vi "Autonomous Independent.vi"   [LabVIEW 2017]
doc: "This VI is called when autonomous begins, and will automatically be terminated when autonomous ends. You can carry out timed or sensor driven robot movement independently without needing to return to the caller."
uses:
  <vilib>/Rock Robotics/WPI/Utilities/WPI_GetSetVariantRefNum.vi
  <vilib>/Rock Robotics/Network Tables/NT Read String.vi
  <vilib>/Rock Robotics/Network Tables/NT Write Numeric Array.vi
  <vilib>/Rock Robotics/WPI/RobotDrive/WPI_RobotDriveArcadeDrive_Standard(NoSaturation).vi
panel:
  # "Be sure to right-click and choose Data Operations>>Make Current Value default if you want to save the array values with the VI"
types:
  T1 = typedef "WPI_JoystickDevRef.ctl" = cluster{"Device":T2}
  T2 = typedef "WPI_JoystickDeviceEnum.ctl" = enum16{"USB 0", "USB 1", "USB 2", "USB 3", "USB 4", "USB 5"}
  T3 = typedef "WPI_RobotDriveDevRef.ctl" = cluster{"DevStatus":errorcluster, "Motors[]":T4[], "Square Inputs":bool, "Max Output":dbl}
  T4 = typedef "WPI_MotorControlDeviceRef.ctl" = cluster{"DeviceStatus":errorcluster, "Type":T5, "PWM":cluster{"PWM Channel":T6, "DeadBand":T7}, "CAN":cluster{"Device Number":u8, "SetOutput VI Ref":variant, "GetOutput VI Ref":variant, "Enable VI Ref":variant, "Disable VI Ref":variant, "Data":variant}, "Invert":bool, "DIO PWM":cluster{"PWM \"Enable\" Channel":T6, "DIOChannel":T8, "PWM Rate":dbl}}
  T5 = typedef "WPI_MotorControlType.ctl" = enum16{"PWM", "CAN", "DIO PWM"}
  T6 = typedef "FPGA_DIOPWMChannel.ctl" = enum8{"PWM 0", "PWM 1", "PWM 2", "PWM 3", "PWM 4", "PWM 5", "PWM 6", "PWM 7", "PWM 8", "PWM 9", "PWM MXP 0", "PWM MXP 1", "PWM MXP 2", "PWM MXP 3", "PWM MXP 4", "PWM MXP 5", "PWM MXP 6", "PWM MXP 7", "PWM MXP 8", "PWM MXP 9", "Invalid"}
  T7 = typedef "WPI_PWMDeadband.ctl" = cluster{"Name":string, "maxPositivePwm":i32, "minPositivePwm":i32, "centerPwm":i32, "maxNegativePwm":i32, "minNegativePwm":i32, "angularRange":u16}
  T8 = typedef "FPGA_DIOChannel.ctl" = enum8{"DIO 0", "DIO 1", "DIO 2", "DIO 3", "DIO 4", "DIO 5", "DIO 6", "DIO 7", "DIO 8", "DIO 9", "DIO MXP 0", "DIO MXP 1", "DIO MXP 2", "DIO MXP 3", "DIO MXP 4", "DIO MXP 5", "DIO MXP 6", "DIO MXP 7", "DIO MXP 8", "DIO MXP 9", "DIO MXP 10", "DIO MXP 11", "DIO MXP 12", "DIO MXP 13", "DIO MXP 14", "DIO MXP 15", "SPI Port CS1", "SPI Port CS2", "SPI Port CS3", "SPI Port MISO", "SPI Port MOSI", "Invalid"}
  T9 = typedef "WPI_SwitchDevRef.ctl" = cluster{"DevStatus":errorcluster, "DIO Channel":T8, "CntIndex":T10, "Normally Closed":bool}
  T10 = typedef "FPGA_CounterCtrSystemIndex.ctl" = enum8{"Ctr 0", "Ctr 1", "Ctr 2", "Ctr 3", "Ctr 4", "Ctr 5", "Ctr 6", "Ctr 7", "Invalid"}
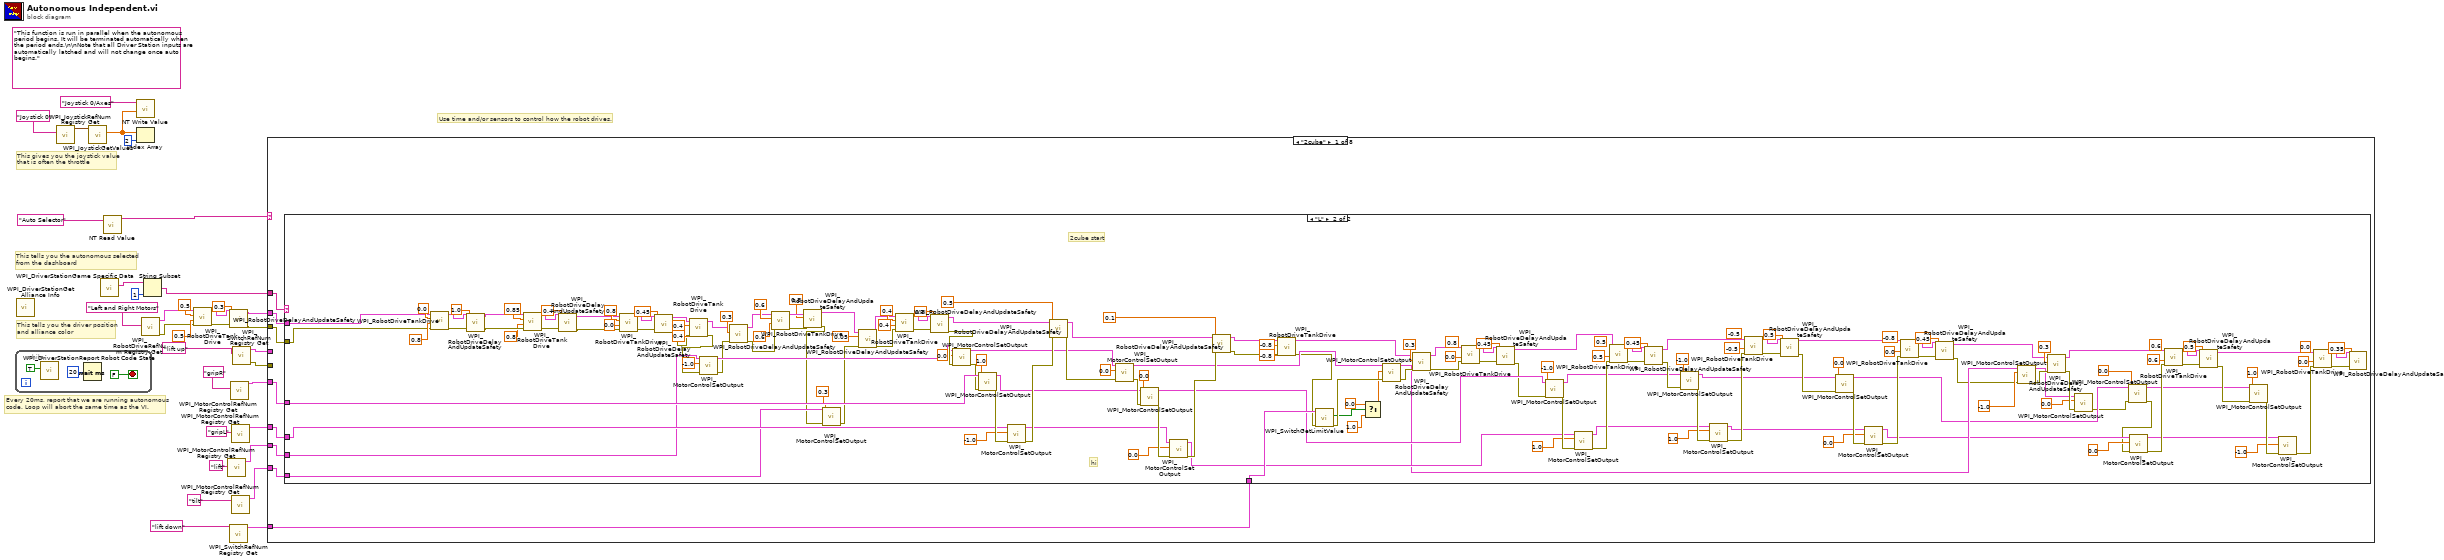
[diagram p0: block diagram]
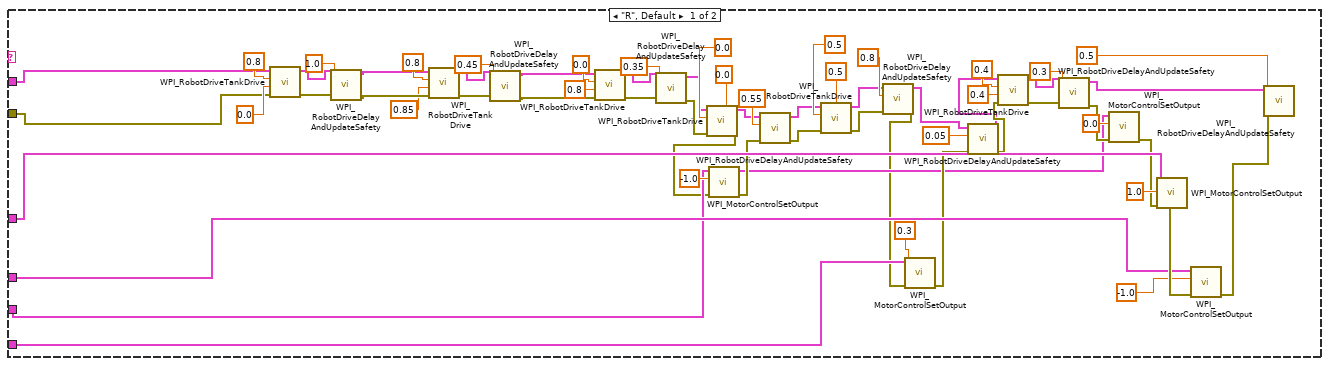
[diagram p2: hidden frame]
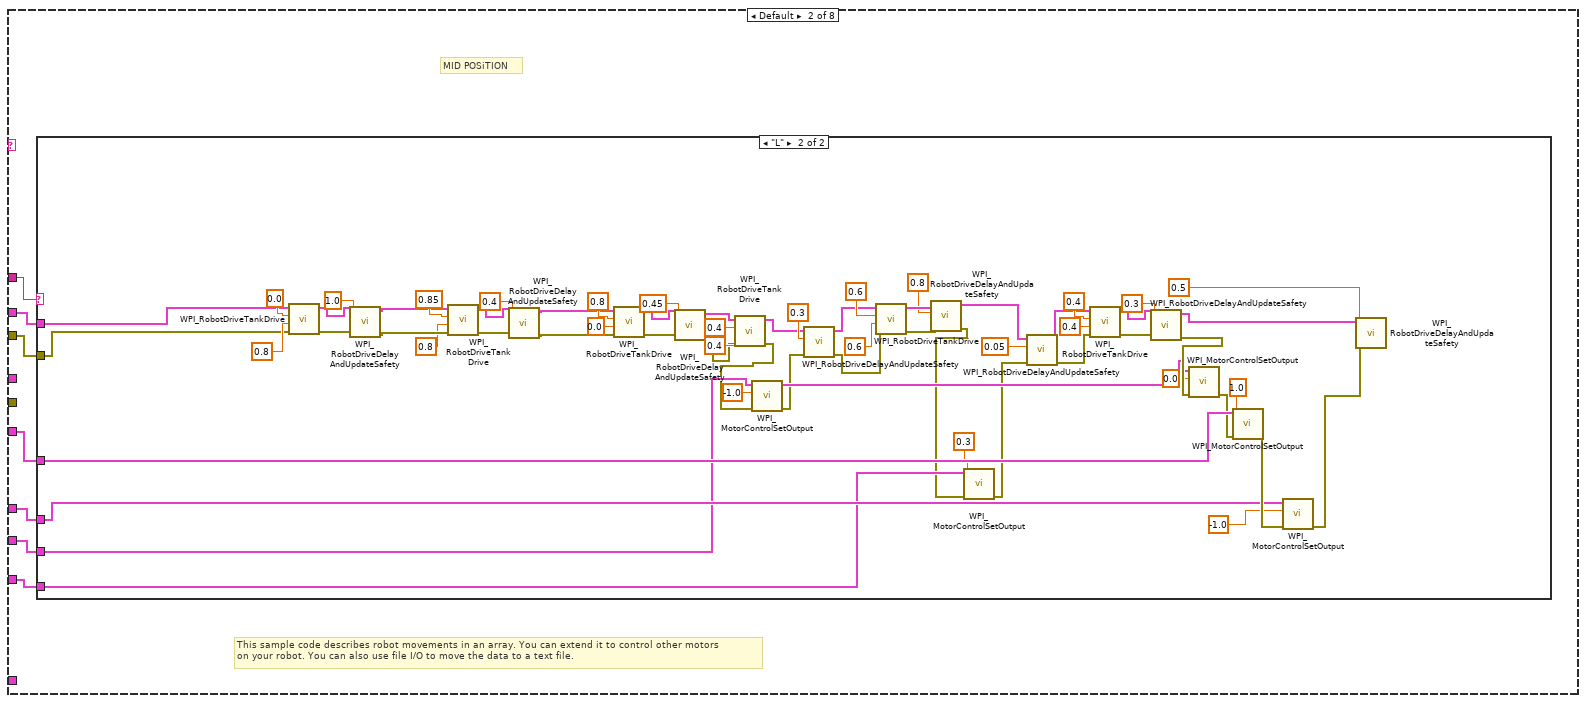
[diagram p3: hidden frame]
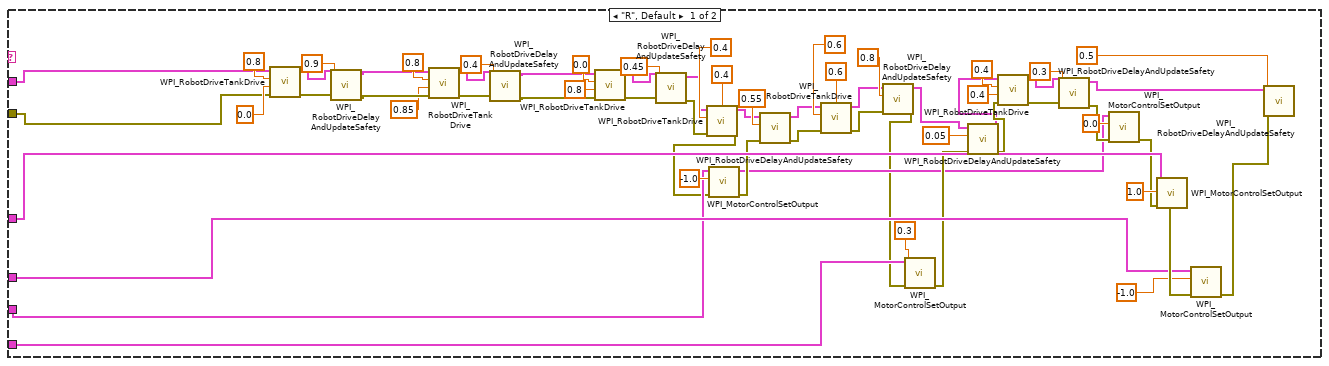
[diagram p4: hidden frame]
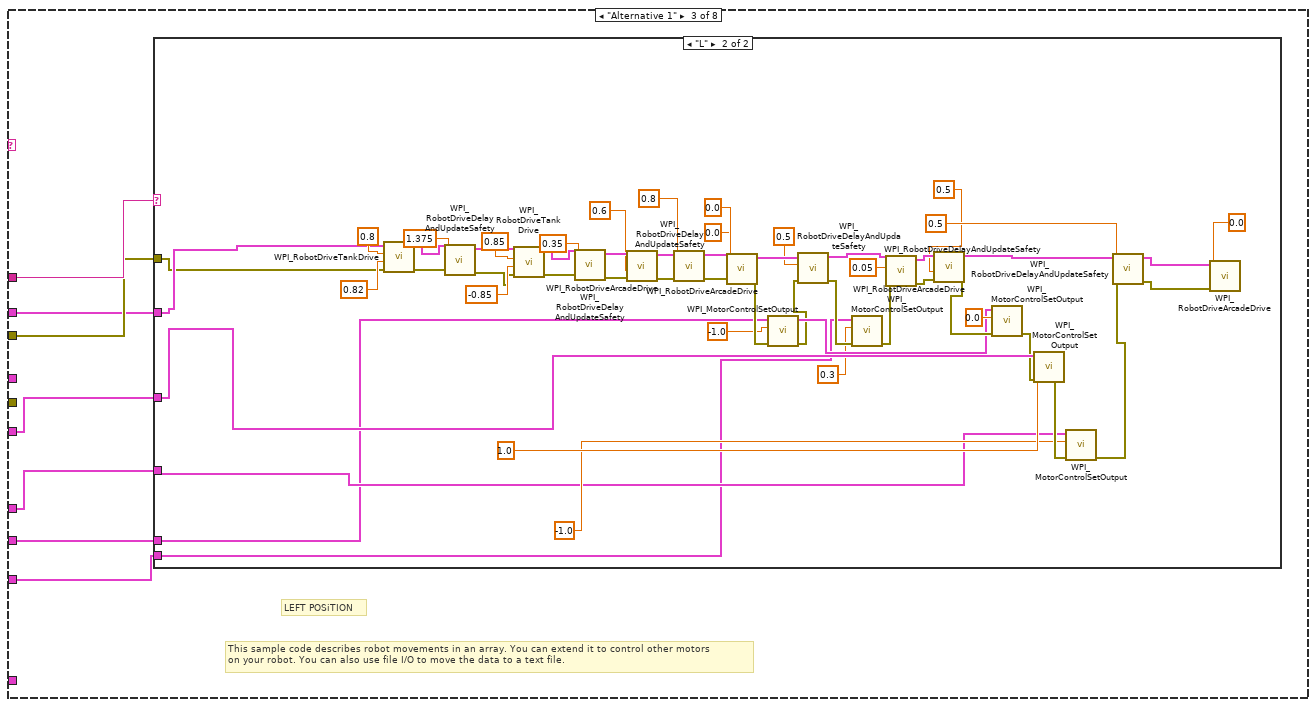
[diagram p5: hidden frame]
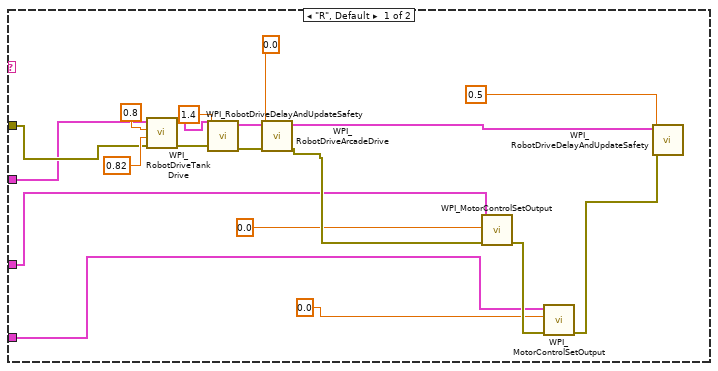
[diagram p6: hidden frame]
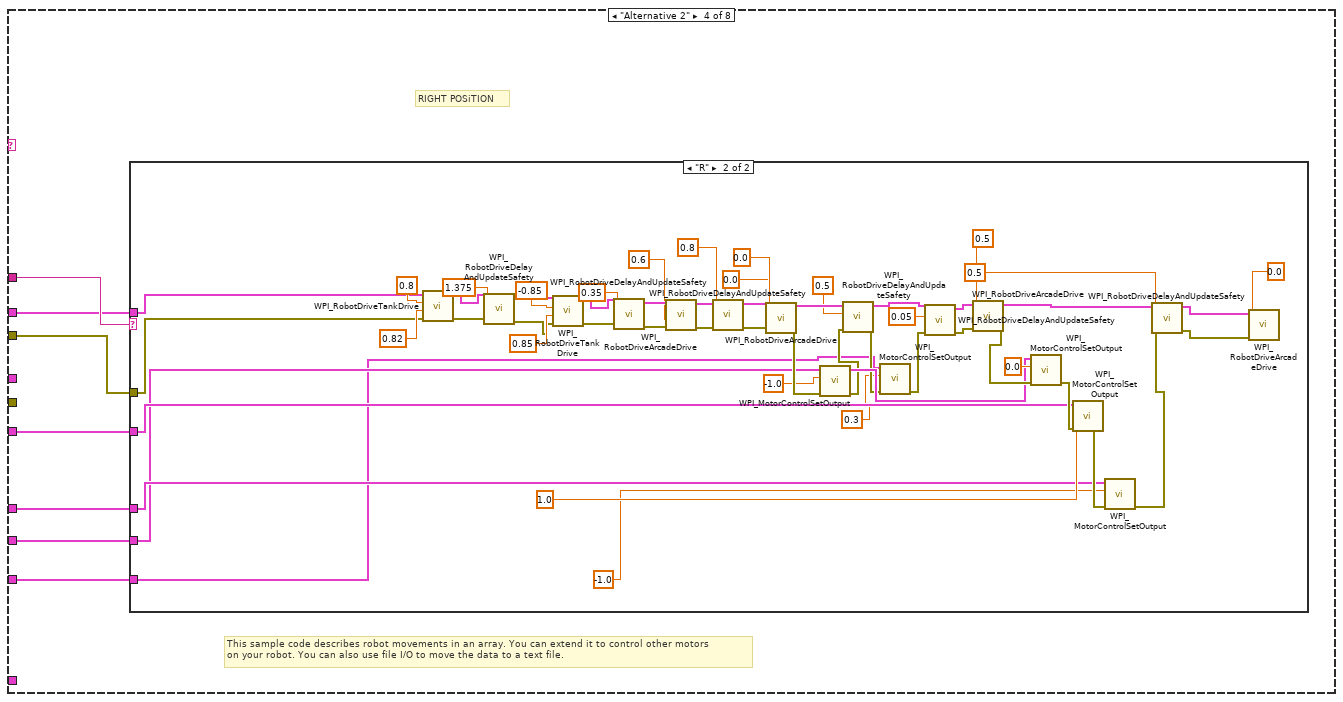
[diagram p7: hidden frame]
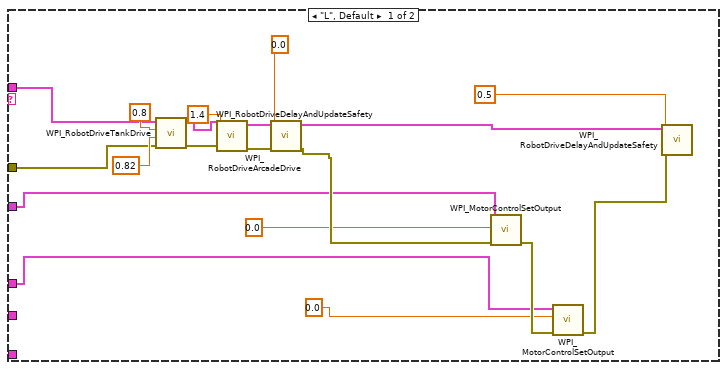
[diagram p8: hidden frame]
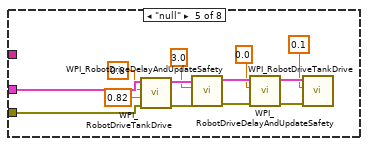
[diagram p9: hidden frame]
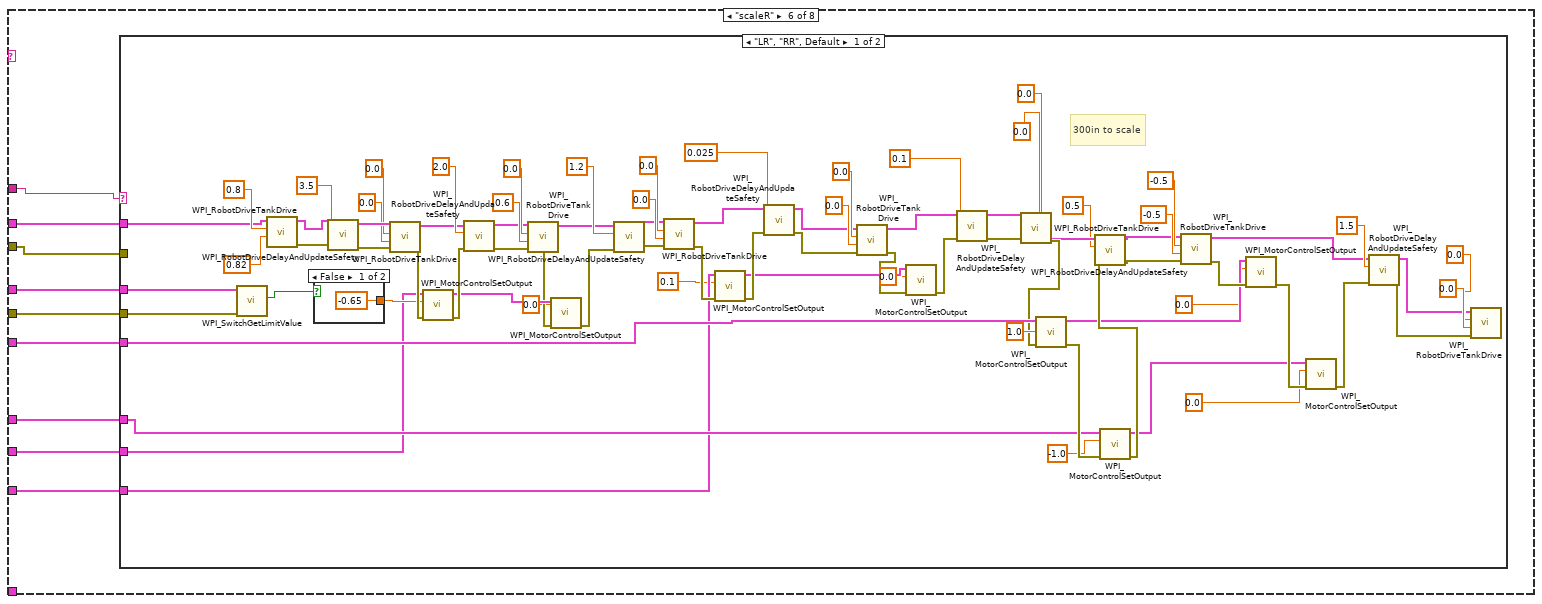
[diagram p10: hidden frame]
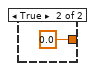
[diagram p11: hidden frame]
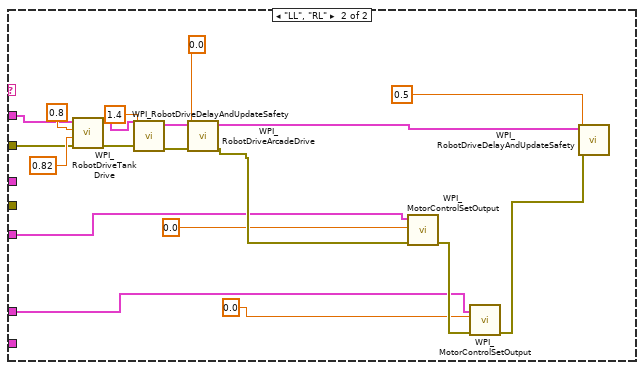
[diagram p12: hidden frame]
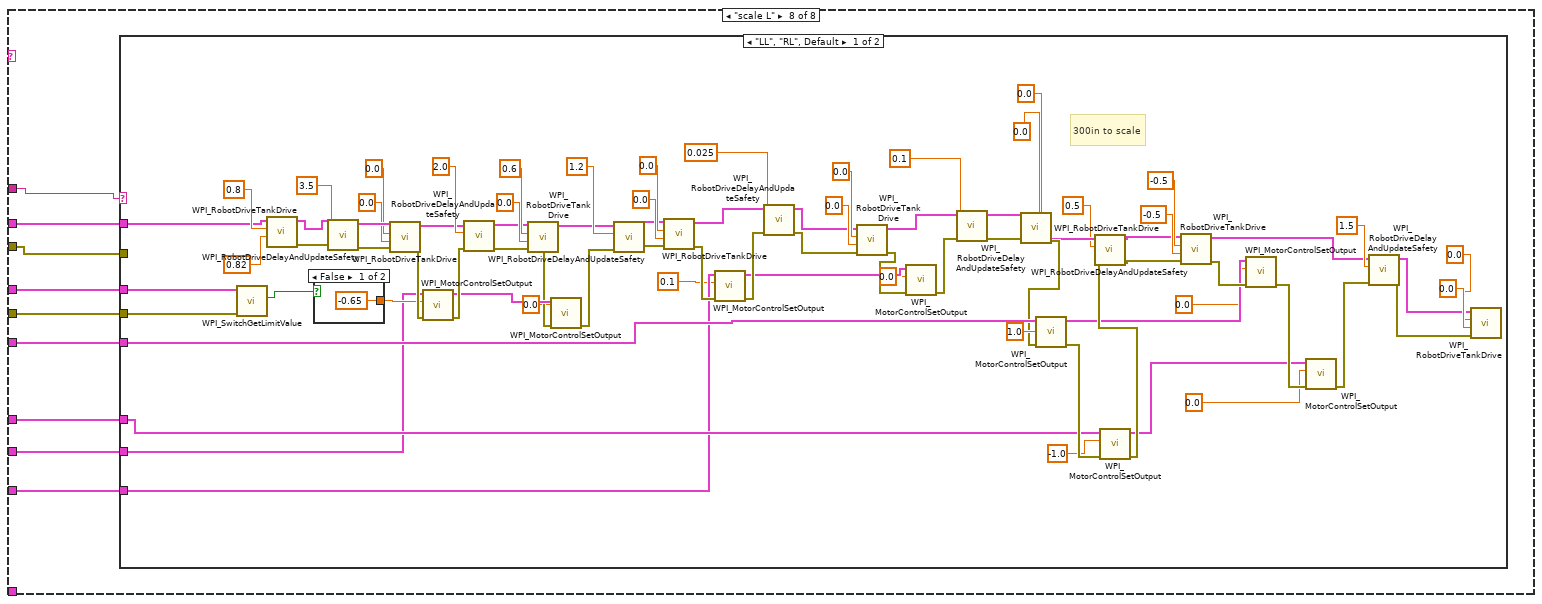
[diagram p14: hidden frame]
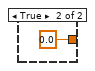
[diagram p15: hidden frame]
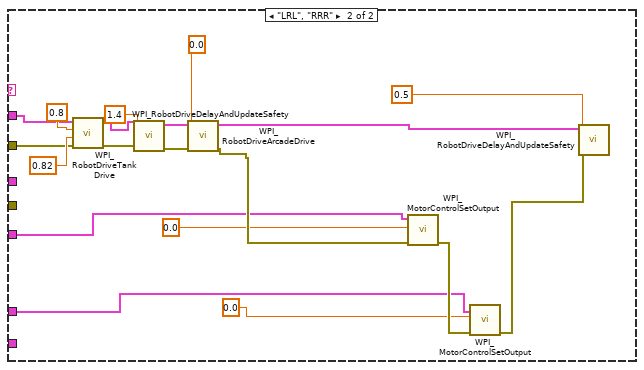
[diagram p16: hidden frame]
diagram:
  (unwired) "This function is run in parallel when the autonomous period begins. It will be terminated automatically when the period ends.\n\nNote that all Driver Station inputs are automatically latched and will not change once auto begins."
  # "This tells you the autonomous selected\nfrom the dashboard"
  # "Every 20ms, report that we are running autonomous\ncode. Loop will abort the same time as the VI."
  # "This gives you the joystick value\nthat is often the throttle"
  # "Use time and/or sensors to control how the robot drives."
  # "This tells you the driver position\nand alliance color"
  n1 = while {
    stop <- FALSE stop-if-true
    n2 = call <vilib>:"WPI_DriverStationReport Robot Code State.vi"("Autonomous"=TRUE) -> ()  [unwired: 10 in, 1 out]
    n3 = Wait (ms)(milliseconds to wait=u32 20) -> ()  [unwired: 1 out]
  }
  n4 = call <vilib>:"WPI_DriverStationGet Alliance Info.vi"() -> ()  [unwired: 12 out]
  n5 = call <vilib>:"WPI_JoystickRefNum Registry Get.vi"("refnum name"="Joystick 0") -> ("JoystickDevRef"=w32:T1)  [unwired: 1 in, 9 out]
  n6 = call <vilib>:"WPI_JoystickGetValues.vi"("JoystickDevRef"=w32) -> ("Axes"=w28:dbl[])  [unwired: 6 in, 4 out]
  n7 = call <vilib>:"WPI_DriverStationGame Specific Data.vi"() -> ("Game Specific Data"=w26:string)  [unwired: 11 in]
  n8 = call-poly <vilib>:"NT Read Value.vi"("Name"="Auto Selector") -> ("String"=w29:string)  [unwired: 9 in, 1 out]
  n9 = call-poly <vilib>:"NT Write Value.vi"("Numeric Array"=w28, "Name"="Joystick 0/Axes") -> ()  [unwired: 9 in, 1 out]
  n10 = Index Array(array=w28, index=2) -> ()  [unwired: 1 out]
  n11 = call <vilib>:"WPI_RobotDriveRefNum Registry Get.vi"("refnum name"="Left and Right Motors") -> ("error out"=w8:errorcluster, "RobotDriveDevRef"=w7:T3)  [unwired: 1 in, 8 out]
  n12 = String Subset(string=w26, length (rest)=1 ("length (rest)")) -> (substring=w24:string)  [unwired: 1 in]
  n13 = call <vilib>:"WPI_RobotDriveTankDrive.vi"("error in (no error)"=w8, "Right axis value"=0.5 ("Y axis value"), "Left axis value"=0.5 ("X axis value"), "RobotDriveDevRef"=w7) -> ("error out"=w12:errorcluster, "RobotDriveDevRef"=w11:T3)  [unwired: 5 in, 1 out]
  n14 = call <vilib>:"WPI_MotorControlRefNum Registry Get.vi"("refnum name"="lift") -> ("MotorControlDevRef"=w14:T4)  [unwired: 9 in, 1 out]
  n15 = call <vilib>:"WPI_RobotDriveDelayAndUpdateSafety.vi"("error in (no error)"=w12, "Delay (s)"=0.3, "RobotDriveDevRef"=w11) -> ("error out"=w5:errorcluster, "RobotDriveDevRef 2"=w6:T3)  [unwired: 7 in]
  n16 = call <vilib>:"WPI_SwitchRefNum Registry Get.vi"("refnum name"="lift down") -> ("SwitchDevRef"=w1:T9)  [unwired: 9 in, 1 out]
  n17 = call <vilib>:"WPI_MotorControlRefNum Registry Get.vi"("refnum name"="gripR") -> ("MotorControlDevRef"=w21:T4)  [unwired: 9 in, 1 out]
  n18 = call <vilib>:"WPI_MotorControlRefNum Registry Get.vi"("refnum name"="gripL") -> ("MotorControlDevRef"=w19:T4)  [unwired: 9 in, 1 out]
  n19 = call <vilib>:"WPI_MotorControlRefNum Registry Get.vi"("refnum name"="tilt") -> ("MotorControlDevRef"=w4:T4)  [unwired: 9 in, 1 out]
  n20 = call <vilib>:"WPI_SwitchRefNum Registry Get.vi"("refnum name"="lift up") -> ("error out"=w16:errorcluster, "SwitchDevRef"=w15:T9)  [unwired: 9 in]
  n21 = case shown="\"2cube\"" w29 {
    tunnel: w24 -> [w44 w279 w412 w492 _ w587 _ w696]
    tunnel: w5 -> [w42 w278 w411 w491 w575 w580 _ w689]
    tunnel: w21 -> [w41 w277 w410 w490 _ w584 _ w693]
    tunnel: w19 -> [w40 w276 w409 w489 _ w585 _ w694]
    tunnel: w6 -> [w43 w275 w408 w488 w576 w586 _ w695]
    tunnel: w16 -> [_ _ _ _ _ w583 _ w692]
    tunnel: w15 -> [_ _ _ _ _ w582 _ w691]
    tunnel: w14 -> [w39 w274 w407 w487 _ w581 _ w690]
    tunnel: w4 -> [w38 w273 w406 w486 _ w579 _ w688]
    tunnel: w1 -> [w37 _ _ _ _ _ _ _]
    frame "2cube" {
      n22 = case shown="\"L\"" w44 {
        tunnel: w42 -> [w97 w242]
        tunnel: w41 -> [w96 w241]
        tunnel: w40 -> [w95 w240]
        tunnel: w43 -> [w74 w239]
        tunnel: w39 -> [w64 w234]
        tunnel: w38 -> [w63 w229]
        tunnel: w37 -> [_ w189]
        frame "R", Default {
          n23 = call <vilib>:"WPI_RobotDriveTankDrive.vi"("error in (no error)"=w97, "Right axis value"=0.0 ("Y axis value"), "Left axis value"=0.8 ("X axis value"), "RobotDriveDevRef"=w74) -> ("error out"=w103:errorcluster, "RobotDriveDevRef"=w102:T3)  [unwired: 5 in, 1 out]
          n24 = call <vilib>:"WPI_RobotDriveDelayAndUpdateSafety.vi"("error in (no error)"=w103, "Delay (s)"=1.0, "RobotDriveDevRef"=w102) -> ("error out"=w89:errorcluster, "RobotDriveDevRef 2"=w90:T3)  [unwired: 7 in]
          n25 = call <vilib>:"WPI_RobotDriveTankDrive.vi"("error in (no error)"=w89, "Right axis value"=0.85, "Left axis value"=0.8 ("X axis value"), "RobotDriveDevRef"=w90) -> ("error out"=w93:errorcluster, "RobotDriveDevRef"=w92:T3)  [unwired: 5 in, 1 out]
          n26 = call <vilib>:"WPI_RobotDriveDelayAndUpdateSafety.vi"("error in (no error)"=w93, "Delay (s)"=0.45, "RobotDriveDevRef"=w92) -> ("error out"=w82:errorcluster, "RobotDriveDevRef 2"=w83:T3)  [unwired: 7 in]
          n27 = call <vilib>:"WPI_RobotDriveTankDrive.vi"("error in (no error)"=w82, "Right axis value"=0.8, "Left axis value"=0.0 ("X axis value"), "RobotDriveDevRef"=w83) -> ("error out"=w86:errorcluster, "RobotDriveDevRef"=w85:T3)  [unwired: 5 in, 1 out]
          n28 = call <vilib>:"WPI_RobotDriveDelayAndUpdateSafety.vi"("error in (no error)"=w86, "Delay (s)"=0.35, "RobotDriveDevRef"=w85) -> ("error out"=w51:errorcluster, "RobotDriveDevRef 2"=w52:T3)  [unwired: 7 in]
          n29 = call <vilib>:"WPI_RobotDriveTankDrive.vi"("error in (no error)"=w51, "Right axis value"=0.0 ("Y axis value"), "Left axis value"=0.0 ("X axis value"), "RobotDriveDevRef"=w52) -> ("error out"=w50:errorcluster, "RobotDriveDevRef"=w49:T3)  [unwired: 5 in, 1 out]
          n30 = call <vilib>:"WPI_MotorControlSetOutput.vi"("error in (no error)"=w50, "Output"=-1.0, "MotorControlDevRef"=w64) -> ("error out"=w67:errorcluster, "MotorControlDevRef"=w62:T4)  [unwired: 6 in, 1 out]
          n31 = call <vilib>:"WPI_RobotDriveDelayAndUpdateSafety.vi"("error in (no error)"=w67, "Delay (s)"=0.55 ("Output"), "RobotDriveDevRef"=w49) -> ("error out"=w48:errorcluster, "RobotDriveDevRef 2"=w47:T3)  [unwired: 7 in]
          n32 = call <vilib>:"WPI_RobotDriveTankDrive.vi"("error in (no error)"=w48, "Right axis value"=0.5 ("Y axis value"), "Left axis value"=0.5 ("X axis value"), "RobotDriveDevRef"=w47) -> ("error out"=w57:errorcluster, "RobotDriveDevRef"=w58:T3)  [unwired: 5 in, 1 out]
          n33 = call <vilib>:"WPI_RobotDriveDelayAndUpdateSafety.vi"("error in (no error)"=w57, "Delay (s)"=0.8, "RobotDriveDevRef"=w58) -> ("error out"=w45:errorcluster, "RobotDriveDevRef 2"=w46:T3)  [unwired: 7 in]
          n34 = call <vilib>:"WPI_MotorControlSetOutput.vi"("error in (no error)"=w45, "Output"=0.3, "MotorControlDevRef"=w63) -> ("error out"=w66:errorcluster)  [unwired: 6 in, 2 out]
          n35 = call <vilib>:"WPI_RobotDriveDelayAndUpdateSafety.vi"("error in (no error)"=w66, "Delay (s)"=0.05, "RobotDriveDevRef"=w46) -> ("error out"=w65:errorcluster, "RobotDriveDevRef 2"=w61:T3)  [unwired: 7 in]
          n36 = call <vilib>:"WPI_RobotDriveTankDrive.vi"("error in (no error)"=w65, "Right axis value"=0.4, "Left axis value"=0.4 ("X axis value"), "RobotDriveDevRef"=w61) -> ("error out"=w79:errorcluster, "RobotDriveDevRef"=w78:T3)  [unwired: 5 in, 1 out]
          n37 = call <vilib>:"WPI_RobotDriveDelayAndUpdateSafety.vi"("error in (no error)"=w79, "Delay (s)"=0.3, "RobotDriveDevRef"=w78) -> ("error out"=w73:errorcluster, "RobotDriveDevRef 2"=w75:T3)  [unwired: 7 in]
          n38 = call <vilib>:"WPI_MotorControlSetOutput.vi"("error in (no error)"=w73, "Output"=0.0, "MotorControlDevRef"=w62) -> ("error out"=w71:errorcluster)  [unwired: 6 in, 2 out]
          n39 = call <vilib>:"WPI_MotorControlSetOutput.vi"("error in (no error)"=w71, "Output"=1.0, "MotorControlDevRef"=w96) -> ("error out"=w105:errorcluster)  [unwired: 6 in, 2 out]
          n40 = call <vilib>:"WPI_MotorControlSetOutput.vi"("error in (no error)"=w105, "Output"=-1.0, "MotorControlDevRef"=w95) -> ("error out"=w104:errorcluster)  [unwired: 6 in, 2 out]
          n41 = call <vilib>:"WPI_RobotDriveDelayAndUpdateSafety.vi"("error in (no error)"=w104, "Delay (s)"=0.5, "RobotDriveDevRef"=w75) -> ()  [unwired: 7 in, 2 out]
        }
        frame "L" {
          (unwired) 0.0 ("X axis value")
          (unwired) 0.6 ("X axis value")
          (unwired) -0.8 ("X axis value")
          (unwired) -0.5 ("X axis value")
          (unwired) 0.5 ("X axis value")
          (unwired) 0.8 ("X axis value")
          # "hi"
          # "2cube start"
          n42 = call <vilib>:"WPI_RobotDriveTankDrive.vi"("error in (no error)"=w242, "Right axis value"=0.8 ("Y axis value"), "Left axis value"=0.0 ("X axis value"), "RobotDriveDevRef"=w239) -> ("error out"=w268:errorcluster, "RobotDriveDevRef"=w267:T3)  [unwired: 5 in, 1 out]
          n43 = call <vilib>:"WPI_RobotDriveDelayAndUpdateSafety.vi"("error in (no error)"=w268, "Delay (s)"=1.0, "RobotDriveDevRef"=w267) -> ("error out"=w257:errorcluster, "RobotDriveDevRef 2"=w258:T3)  [unwired: 7 in]
          n44 = call <vilib>:"WPI_RobotDriveTankDrive.vi"("error in (no error)"=w257, "Right axis value"=0.8, "Left axis value"=0.85 ("X axis value"), "RobotDriveDevRef"=w258) -> ("error out"=w261:errorcluster, "RobotDriveDevRef"=w260:T3)  [unwired: 5 in, 1 out]
          n45 = call <vilib>:"WPI_RobotDriveDelayAndUpdateSafety.vi"("error in (no error)"=w261, "Delay (s)"=0.4, "RobotDriveDevRef"=w260) -> ("error out"=w250:errorcluster, "RobotDriveDevRef 2"=w251:T3)  [unwired: 7 in]
          n46 = call <vilib>:"WPI_RobotDriveTankDrive.vi"("error in (no error)"=w250, "Right axis value"=0.0, "Left axis value"=0.8 ("X axis value"), "RobotDriveDevRef"=w251) -> ("error out"=w254:errorcluster, "RobotDriveDevRef"=w253:T3)  [unwired: 5 in, 1 out]
          n47 = call <vilib>:"WPI_RobotDriveDelayAndUpdateSafety.vi"("error in (no error)"=w254, "Delay (s)"=0.45, "RobotDriveDevRef"=w253) -> ("error out"=w216:errorcluster, "RobotDriveDevRef 2"=w217:T3)  [unwired: 7 in]
          n48 = call <vilib>:"WPI_RobotDriveTankDrive.vi"("error in (no error)"=w216, "Right axis value"=0.4, "Left axis value"=0.4, "RobotDriveDevRef"=w217) -> ("error out"=w214:errorcluster, "RobotDriveDevRef"=w215:T3)  [unwired: 5 in, 1 out]
          n49 = call <vilib>:"WPI_MotorControlSetOutput.vi"("error in (no error)"=w214, "Output"=-1.0, "MotorControlDevRef"=w234) -> ("error out"=w227:errorcluster, "MotorControlDevRef"=w231:T4)  [unwired: 6 in, 1 out]
          n50 = call <vilib>:"WPI_RobotDriveDelayAndUpdateSafety.vi"("error in (no error)"=w227, "Delay (s)"=0.3 ("Output"), "RobotDriveDevRef"=w215) -> ("error out"=w211:errorcluster, "RobotDriveDevRef 2"=w213:T3)  [unwired: 7 in]
          n51 = call <vilib>:"WPI_RobotDriveTankDrive.vi"("error in (no error)"=w211, "Right axis value"=0.6 ("X axis value"), "Left axis value"=0.6 ("X axis value"), "RobotDriveDevRef"=w213) -> ("error out"=w223:errorcluster, "RobotDriveDevRef"=w224:T3)  [unwired: 5 in, 1 out]
          n52 = call <vilib>:"WPI_RobotDriveDelayAndUpdateSafety.vi"("error in (no error)"=w223, "Delay (s)"=0.8 ("X axis value"), "RobotDriveDevRef"=w224) -> ("error out"=w210:errorcluster, "RobotDriveDevRef 2"=w212:T3)  [unwired: 7 in]
          n53 = call <vilib>:"WPI_MotorControlSetOutput.vi"("error in (no error)"=w210, "Output"=0.3, "MotorControlDevRef"=w229) -> ("error out"=w226:errorcluster)  [unwired: 6 in, 2 out]
          n54 = call <vilib>:"WPI_RobotDriveDelayAndUpdateSafety.vi"("error in (no error)"=w226, "Delay (s)"=0.05, "RobotDriveDevRef"=w212) -> ("error out"=w235:errorcluster, "RobotDriveDevRef 2"=w236:T3)  [unwired: 7 in]
          n55 = call <vilib>:"WPI_RobotDriveTankDrive.vi"("error in (no error)"=w235, "Right axis value"=0.4, "Left axis value"=0.4 ("X axis value"), "RobotDriveDevRef"=w236) -> ("error out"=w247:errorcluster, "RobotDriveDevRef"=w246:T3)  [unwired: 5 in, 1 out]
          n56 = call <vilib>:"WPI_RobotDriveDelayAndUpdateSafety.vi"("error in (no error)"=w247, "Delay (s)"=0.3, "RobotDriveDevRef"=w246) -> ("error out"=w233:errorcluster, "RobotDriveDevRef 2"=w243:T3)  [unwired: 7 in]
          n57 = call <vilib>:"WPI_MotorControlSetOutput.vi"("error in (no error)"=w233, "Output"=0.0, "MotorControlDevRef"=w231) -> ("error out"=w232:errorcluster, "MotorControlDevRef"=w200:T4)  [unwired: 6 in, 1 out]
          n58 = call <vilib>:"WPI_MotorControlSetOutput.vi"("error in (no error)"=w232, "Output"=1.0, "MotorControlDevRef"=w241) -> ("error out"=w270:errorcluster, "MotorControlDevRef"=w199:T4)  [unwired: 6 in, 1 out]
          n59 = call <vilib>:"WPI_MotorControlSetOutput.vi"("error in (no error)"=w270, "Output"=-1.0, "MotorControlDevRef"=w240) -> ("error out"=w269:errorcluster, "MotorControlDevRef"=w198:T4)  [unwired: 6 in, 1 out]
          n60 = call <vilib>:"WPI_RobotDriveDelayAndUpdateSafety.vi"("error in (no error)"=w269, "Delay (s)"=0.5, "RobotDriveDevRef"=w243) -> ("error out"=w202:errorcluster, "RobotDriveDevRef 2"=w203:T3)  [unwired: 7 in]
          n61 = call <vilib>:"WPI_MotorControlSetOutput.vi"("error in (no error)"=w202, "Output"=0.0, "MotorControlDevRef"=w200) -> ("error out"=w204:errorcluster, "MotorControlDevRef"=w190:T4)  [unwired: 6 in, 1 out]
          n62 = call <vilib>:"WPI_MotorControlSetOutput.vi"("error in (no error)"=w204, "Output"=0.0, "MotorControlDevRef"=w199) -> ("error out"=w208:errorcluster, "MotorControlDevRef"=w169:T4)  [unwired: 6 in, 1 out]
          n63 = call <vilib>:"WPI_MotorControlSetOutput.vi"("error in (no error)"=w208, "Output"=0.0, "MotorControlDevRef"=w198) -> ("error out"=w207:errorcluster, "MotorControlDevRef"=w168:T4)  [unwired: 6 in, 1 out]
          n64 = call <vilib>:"WPI_RobotDriveDelayAndUpdateSafety.vi"("error in (no error)"=w207, "Delay (s)"=0.1, "RobotDriveDevRef"=w203) -> ("error out"=w191:errorcluster, "RobotDriveDevRef 2"=w192:T3)  [unwired: 7 in]
          n65 = call <vilib>:"WPI_RobotDriveTankDrive.vi"("error in (no error)"=w191, "Right axis value"=-0.8, "Left axis value"=-0.8, "RobotDriveDevRef"=w192) -> ("error out"=w188:errorcluster, "RobotDriveDevRef"=w193:T3)  [unwired: 5 in, 1 out]
          n66 = call <vilib>:"WPI_SwitchGetLimitValue.vi"("error in (no error)"=w188, "SwitchDevRef"=w189) -> ("error out"=w187:errorcluster, "Switch Pressed"=w186:bool)  [unwired: 7 in, 1 out]
          n67 = Select(t=0.0, s=w186, f=1.0 ("Output")) -> (s? t:f=w183:dbl)
          n68 = call <vilib>:"WPI_MotorControlSetOutput.vi"("error in (no error)"=w187, "Output"=w183, "MotorControlDevRef"=w190) -> ("error out"=w197:errorcluster, "MotorControlDevRef"=w137:T4)  [unwired: 6 in, 1 out]
          n69 = call <vilib>:"WPI_RobotDriveDelayAndUpdateSafety.vi"("error in (no error)"=w197, "Delay (s)"=0.3 ("Output"), "RobotDriveDevRef"=w193) -> ("error out"=w177:errorcluster, "RobotDriveDevRef 2"=w178:T3)  [unwired: 7 in]
          n70 = call <vilib>:"WPI_RobotDriveTankDrive.vi"("error in (no error)"=w177, "Right axis value"=0.0, "RobotDriveDevRef"=w178) -> ("error out"=w181:errorcluster, "RobotDriveDevRef"=w180:T3)  [unwired: 6 in, 1 out]
          n71 = call <vilib>:"WPI_RobotDriveDelayAndUpdateSafety.vi"("error in (no error)"=w181, "Delay (s)"=0.45, "RobotDriveDevRef"=w180) -> ("error out"=w167:errorcluster, "RobotDriveDevRef 2"=w165:T3)  [unwired: 7 in]
          n72 = call <vilib>:"WPI_MotorControlSetOutput.vi"("error in (no error)"=w167, "Output"=-1.0, "MotorControlDevRef"=w169) -> ("error out"=w172:errorcluster, "MotorControlDevRef"=w142:T4)  [unwired: 6 in, 1 out]
          n73 = call <vilib>:"WPI_MotorControlSetOutput.vi"("error in (no error)"=w172, "Output"=1.0, "MotorControlDevRef"=w168) -> ("error out"=w166:errorcluster, "MotorControlDevRef"=w141:T4)  [unwired: 6 in, 1 out]
          n74 = call <vilib>:"WPI_RobotDriveTankDrive.vi"("error in (no error)"=w166, "Right axis value"=0.5, "RobotDriveDevRef"=w165) -> ("error out"=w175:errorcluster, "RobotDriveDevRef"=w174:T3)  [unwired: 6 in, 1 out]
          n75 = call <vilib>:"WPI_RobotDriveDelayAndUpdateSafety.vi"("error in (no error)"=w175, "Delay (s)"=0.45, "RobotDriveDevRef"=w174) -> ("error out"=w155:errorcluster, "RobotDriveDevRef 2"=w156:T3)  [unwired: 7 in]
          n76 = call <vilib>:"WPI_MotorControlSetOutput.vi"("error in (no error)"=w155, "Output"=-1.0, "MotorControlDevRef"=w142) -> ("error out"=w160:errorcluster, "MotorControlDevRef"=w140:T4)  [unwired: 6 in, 1 out]
          n77 = call <vilib>:"WPI_MotorControlSetOutput.vi"("error in (no error)"=w160, "Output"=1.0, "MotorControlDevRef"=w141) -> ("error out"=w157:errorcluster, "MotorControlDevRef"=w139:T4)  [unwired: 6 in, 1 out]
          n78 = call <vilib>:"WPI_RobotDriveTankDrive.vi"("error in (no error)"=w157, "Right axis value"=-0.5, "RobotDriveDevRef"=w156) -> ("error out"=w163:errorcluster, "RobotDriveDevRef"=w162:T3)  [unwired: 6 in, 1 out]
          n79 = call <vilib>:"WPI_RobotDriveDelayAndUpdateSafety.vi"("error in (no error)"=w163, "Delay (s)"=0.5, "RobotDriveDevRef"=w162) -> ("error out"=w145:errorcluster, "RobotDriveDevRef 2"=w146:T3)  [unwired: 7 in]
          n80 = call <vilib>:"WPI_MotorControlSetOutput.vi"("error in (no error)"=w145, "Output"=0.0, "MotorControlDevRef"=w140) -> ("error out"=w150:errorcluster, "MotorControlDevRef"=w116:T4)  [unwired: 6 in, 1 out]
          n81 = call <vilib>:"WPI_MotorControlSetOutput.vi"("error in (no error)"=w150, "Output"=0.0, "MotorControlDevRef"=w139) -> ("error out"=w147:errorcluster, "MotorControlDevRef"=w114:T4)  [unwired: 6 in, 1 out]
          n82 = call <vilib>:"WPI_RobotDriveTankDrive.vi"("error in (no error)"=w147, "Right axis value"=0.0, "RobotDriveDevRef"=w146) -> ("error out"=w153:errorcluster, "RobotDriveDevRef"=w152:T3)  [unwired: 6 in, 1 out]
          n83 = call <vilib>:"WPI_RobotDriveDelayAndUpdateSafety.vi"("error in (no error)"=w153, "Delay (s)"=0.45, "RobotDriveDevRef"=w152) -> ("error out"=w136:errorcluster, "RobotDriveDevRef 2"=w135:T3)  [unwired: 7 in]
          n84 = call <vilib>:"WPI_MotorControlSetOutput.vi"("error in (no error)"=w136, "Output"=-1.0 ("t"), "MotorControlDevRef"=w137) -> ("error out"=w144:errorcluster, "MotorControlDevRef"=w109:T4)  [unwired: 6 in, 1 out]
          n85 = call <vilib>:"WPI_RobotDriveDelayAndUpdateSafety.vi"("error in (no error)"=w144, "Delay (s)"=0.3 ("Output"), "RobotDriveDevRef"=w135) -> ("error out"=w111:errorcluster, "RobotDriveDevRef 2"=w127:T3)  [unwired: 7 in]
          n86 = call <vilib>:"WPI_MotorControlSetOutput.vi"("error in (no error)"=w111, "Output"=0.0, "MotorControlDevRef"=w109) -> ("error out"=w110:errorcluster)  [unwired: 6 in, 2 out]
          n87 = call <vilib>:"WPI_MotorControlSetOutput.vi"("error in (no error)"=w110, "Output"=0.0, "MotorControlDevRef"=w116) -> ("error out"=w112:errorcluster, "MotorControlDevRef"=w115:T4)  [unwired: 6 in, 1 out]
          n88 = call <vilib>:"WPI_MotorControlSetOutput.vi"("error in (no error)"=w112, "Output"=0.0, "MotorControlDevRef"=w114) -> ("error out"=w128:errorcluster, "MotorControlDevRef"=w113:T4)  [unwired: 6 in, 1 out]
          n89 = call <vilib>:"WPI_RobotDriveTankDrive.vi"("error in (no error)"=w128, "Right axis value"=0.6, "RobotDriveDevRef"=w127) -> ("error out"=w133:errorcluster, "RobotDriveDevRef"=w132:T3)  [unwired: 6 in, 1 out]
          n90 = call <vilib>:"WPI_RobotDriveDelayAndUpdateSafety.vi"("error in (no error)"=w133, "Delay (s)"=0.5, "RobotDriveDevRef"=w132) -> ("error out"=w117:errorcluster, "RobotDriveDevRef 2"=w118:T3)  [unwired: 7 in]
          n91 = call <vilib>:"WPI_MotorControlSetOutput.vi"("error in (no error)"=w117, "Output"=1.0, "MotorControlDevRef"=w115) -> ("error out"=w122:errorcluster)  [unwired: 6 in, 2 out]
          n92 = call <vilib>:"WPI_MotorControlSetOutput.vi"("error in (no error)"=w122, "Output"=-1.0, "MotorControlDevRef"=w113) -> ("error out"=w119:errorcluster)  [unwired: 6 in, 2 out]
          n93 = call <vilib>:"WPI_RobotDriveTankDrive.vi"("error in (no error)"=w119, "Right axis value"=0.0, "RobotDriveDevRef"=w118) -> ("error out"=w125:errorcluster, "RobotDriveDevRef"=w124:T3)  [unwired: 6 in, 1 out]
          n94 = call <vilib>:"WPI_RobotDriveDelayAndUpdateSafety.vi"("error in (no error)"=w125, "Delay (s)"=0.35, "RobotDriveDevRef"=w124) -> ()  [unwired: 7 in, 2 out]
        }
      }
    }
    frame Default {
      # "MID POSiTION"
      # "This sample code describes robot movements in an array. You can extend it to control other motors\non your robot. You can also use file I/O to move the data to a text file."
      n95 = case shown="\"L\"" w279 {
        tunnel: w278 -> [w332 w375]
        tunnel: w277 -> [w331 w374]
        tunnel: w276 -> [w330 w373]
        tunnel: w275 -> [w309 w372]
        tunnel: w274 -> [w299 w367]
        tunnel: w273 -> [w298 w362]
        frame "R", Default {
          n96 = call <vilib>:"WPI_RobotDriveTankDrive.vi"("error in (no error)"=w332, "Right axis value"=0.0 ("Y axis value"), "Left axis value"=0.8 ("X axis value"), "RobotDriveDevRef"=w309) -> ("error out"=w338:errorcluster, "RobotDriveDevRef"=w337:T3)  [unwired: 5 in, 1 out]
          n97 = call <vilib>:"WPI_RobotDriveDelayAndUpdateSafety.vi"("error in (no error)"=w338, "Delay (s)"=0.9, "RobotDriveDevRef"=w337) -> ("error out"=w324:errorcluster, "RobotDriveDevRef 2"=w325:T3)  [unwired: 7 in]
          n98 = call <vilib>:"WPI_RobotDriveTankDrive.vi"("error in (no error)"=w324, "Right axis value"=0.85, "Left axis value"=0.8 ("X axis value"), "RobotDriveDevRef"=w325) -> ("error out"=w328:errorcluster, "RobotDriveDevRef"=w327:T3)  [unwired: 5 in, 1 out]
          n99 = call <vilib>:"WPI_RobotDriveDelayAndUpdateSafety.vi"("error in (no error)"=w328, "Delay (s)"=0.4, "RobotDriveDevRef"=w327) -> ("error out"=w317:errorcluster, "RobotDriveDevRef 2"=w318:T3)  [unwired: 7 in]
          n100 = call <vilib>:"WPI_RobotDriveTankDrive.vi"("error in (no error)"=w317, "Right axis value"=0.8, "Left axis value"=0.0 ("X axis value"), "RobotDriveDevRef"=w318) -> ("error out"=w321:errorcluster, "RobotDriveDevRef"=w320:T3)  [unwired: 5 in, 1 out]
          n101 = call <vilib>:"WPI_RobotDriveDelayAndUpdateSafety.vi"("error in (no error)"=w321, "Delay (s)"=0.45, "RobotDriveDevRef"=w320) -> ("error out"=w286:errorcluster, "RobotDriveDevRef 2"=w287:T3)  [unwired: 7 in]
          n102 = call <vilib>:"WPI_RobotDriveTankDrive.vi"("error in (no error)"=w286, "Right axis value"=0.4 ("Y axis value"), "Left axis value"=0.4 ("X axis value"), "RobotDriveDevRef"=w287) -> ("error out"=w285:errorcluster, "RobotDriveDevRef"=w284:T3)  [unwired: 5 in, 1 out]
          n103 = call <vilib>:"WPI_MotorControlSetOutput.vi"("error in (no error)"=w285, "Output"=-1.0, "MotorControlDevRef"=w299) -> ("error out"=w302:errorcluster, "MotorControlDevRef"=w297:T4)  [unwired: 6 in, 1 out]
          n104 = call <vilib>:"WPI_RobotDriveDelayAndUpdateSafety.vi"("error in (no error)"=w302, "Delay (s)"=0.55 ("Output"), "RobotDriveDevRef"=w284) -> ("error out"=w283:errorcluster, "RobotDriveDevRef 2"=w282:T3)  [unwired: 7 in]
          n105 = call <vilib>:"WPI_RobotDriveTankDrive.vi"("error in (no error)"=w283, "Right axis value"=0.6 ("Y axis value"), "Left axis value"=0.6 ("X axis value"), "RobotDriveDevRef"=w282) -> ("error out"=w292:errorcluster, "RobotDriveDevRef"=w293:T3)  [unwired: 5 in, 1 out]
          n106 = call <vilib>:"WPI_RobotDriveDelayAndUpdateSafety.vi"("error in (no error)"=w292, "Delay (s)"=0.8, "RobotDriveDevRef"=w293) -> ("error out"=w280:errorcluster, "RobotDriveDevRef 2"=w281:T3)  [unwired: 7 in]
          n107 = call <vilib>:"WPI_MotorControlSetOutput.vi"("error in (no error)"=w280, "Output"=0.3, "MotorControlDevRef"=w298) -> ("error out"=w301:errorcluster)  [unwired: 6 in, 2 out]
          n108 = call <vilib>:"WPI_RobotDriveDelayAndUpdateSafety.vi"("error in (no error)"=w301, "Delay (s)"=0.05, "RobotDriveDevRef"=w281) -> ("error out"=w300:errorcluster, "RobotDriveDevRef 2"=w296:T3)  [unwired: 7 in]
          n109 = call <vilib>:"WPI_RobotDriveTankDrive.vi"("error in (no error)"=w300, "Right axis value"=0.4, "Left axis value"=0.4 ("X axis value"), "RobotDriveDevRef"=w296) -> ("error out"=w314:errorcluster, "RobotDriveDevRef"=w313:T3)  [unwired: 5 in, 1 out]
          n110 = call <vilib>:"WPI_RobotDriveDelayAndUpdateSafety.vi"("error in (no error)"=w314, "Delay (s)"=0.3, "RobotDriveDevRef"=w313) -> ("error out"=w308:errorcluster, "RobotDriveDevRef 2"=w310:T3)  [unwired: 7 in]
          n111 = call <vilib>:"WPI_MotorControlSetOutput.vi"("error in (no error)"=w308, "Output"=0.0, "MotorControlDevRef"=w297) -> ("error out"=w306:errorcluster)  [unwired: 6 in, 2 out]
          n112 = call <vilib>:"WPI_MotorControlSetOutput.vi"("error in (no error)"=w306, "Output"=1.0, "MotorControlDevRef"=w331) -> ("error out"=w340:errorcluster)  [unwired: 6 in, 2 out]
          n113 = call <vilib>:"WPI_MotorControlSetOutput.vi"("error in (no error)"=w340, "Output"=-1.0, "MotorControlDevRef"=w330) -> ("error out"=w339:errorcluster)  [unwired: 6 in, 2 out]
          n114 = call <vilib>:"WPI_RobotDriveDelayAndUpdateSafety.vi"("error in (no error)"=w339, "Delay (s)"=0.5, "RobotDriveDevRef"=w310) -> ()  [unwired: 7 in, 2 out]
        }
        frame "L" {
          n115 = call <vilib>:"WPI_RobotDriveTankDrive.vi"("error in (no error)"=w375, "Right axis value"=0.8 ("Y axis value"), "Left axis value"=0.0 ("X axis value"), "RobotDriveDevRef"=w372) -> ("error out"=w401:errorcluster, "RobotDriveDevRef"=w400:T3)  [unwired: 5 in, 1 out]
          n116 = call <vilib>:"WPI_RobotDriveDelayAndUpdateSafety.vi"("error in (no error)"=w401, "Delay (s)"=1.0, "RobotDriveDevRef"=w400) -> ("error out"=w390:errorcluster, "RobotDriveDevRef 2"=w391:T3)  [unwired: 7 in]
          n117 = call <vilib>:"WPI_RobotDriveTankDrive.vi"("error in (no error)"=w390, "Right axis value"=0.8, "Left axis value"=0.85 ("X axis value"), "RobotDriveDevRef"=w391) -> ("error out"=w394:errorcluster, "RobotDriveDevRef"=w393:T3)  [unwired: 5 in, 1 out]
          n118 = call <vilib>:"WPI_RobotDriveDelayAndUpdateSafety.vi"("error in (no error)"=w394, "Delay (s)"=0.4, "RobotDriveDevRef"=w393) -> ("error out"=w383:errorcluster, "RobotDriveDevRef 2"=w384:T3)  [unwired: 7 in]
          n119 = call <vilib>:"WPI_RobotDriveTankDrive.vi"("error in (no error)"=w383, "Right axis value"=0.0, "Left axis value"=0.8 ("X axis value"), "RobotDriveDevRef"=w384) -> ("error out"=w387:errorcluster, "RobotDriveDevRef"=w386:T3)  [unwired: 5 in, 1 out]
          n120 = call <vilib>:"WPI_RobotDriveDelayAndUpdateSafety.vi"("error in (no error)"=w387, "Delay (s)"=0.45, "RobotDriveDevRef"=w386) -> ("error out"=w349:errorcluster, "RobotDriveDevRef 2"=w350:T3)  [unwired: 7 in]
          n121 = call <vilib>:"WPI_RobotDriveTankDrive.vi"("error in (no error)"=w349, "Right axis value"=0.4, "Left axis value"=0.4, "RobotDriveDevRef"=w350) -> ("error out"=w347:errorcluster, "RobotDriveDevRef"=w348:T3)  [unwired: 5 in, 1 out]
          n122 = call <vilib>:"WPI_MotorControlSetOutput.vi"("error in (no error)"=w347, "Output"=-1.0, "MotorControlDevRef"=w367) -> ("error out"=w360:errorcluster, "MotorControlDevRef"=w364:T4)  [unwired: 6 in, 1 out]
          n123 = call <vilib>:"WPI_RobotDriveDelayAndUpdateSafety.vi"("error in (no error)"=w360, "Delay (s)"=0.3 ("Output"), "RobotDriveDevRef"=w348) -> ("error out"=w344:errorcluster, "RobotDriveDevRef 2"=w346:T3)  [unwired: 7 in]
          n124 = call <vilib>:"WPI_RobotDriveTankDrive.vi"("error in (no error)"=w344, "Right axis value"=0.6 ("X axis value"), "Left axis value"=0.6 ("X axis value"), "RobotDriveDevRef"=w346) -> ("error out"=w356:errorcluster, "RobotDriveDevRef"=w357:T3)  [unwired: 5 in, 1 out]
          n125 = call <vilib>:"WPI_RobotDriveDelayAndUpdateSafety.vi"("error in (no error)"=w356, "Delay (s)"=0.8 ("X axis value"), "RobotDriveDevRef"=w357) -> ("error out"=w343:errorcluster, "RobotDriveDevRef 2"=w345:T3)  [unwired: 7 in]
          n126 = call <vilib>:"WPI_MotorControlSetOutput.vi"("error in (no error)"=w343, "Output"=0.3, "MotorControlDevRef"=w362) -> ("error out"=w359:errorcluster)  [unwired: 6 in, 2 out]
          n127 = call <vilib>:"WPI_RobotDriveDelayAndUpdateSafety.vi"("error in (no error)"=w359, "Delay (s)"=0.05, "RobotDriveDevRef"=w345) -> ("error out"=w368:errorcluster, "RobotDriveDevRef 2"=w369:T3)  [unwired: 7 in]
          n128 = call <vilib>:"WPI_RobotDriveTankDrive.vi"("error in (no error)"=w368, "Right axis value"=0.4, "Left axis value"=0.4 ("X axis value"), "RobotDriveDevRef"=w369) -> ("error out"=w380:errorcluster, "RobotDriveDevRef"=w379:T3)  [unwired: 5 in, 1 out]
          n129 = call <vilib>:"WPI_RobotDriveDelayAndUpdateSafety.vi"("error in (no error)"=w380, "Delay (s)"=0.3, "RobotDriveDevRef"=w379) -> ("error out"=w366:errorcluster, "RobotDriveDevRef 2"=w376:T3)  [unwired: 7 in]
          n130 = call <vilib>:"WPI_MotorControlSetOutput.vi"("error in (no error)"=w366, "Output"=0.0, "MotorControlDevRef"=w364) -> ("error out"=w365:errorcluster)  [unwired: 6 in, 2 out]
          n131 = call <vilib>:"WPI_MotorControlSetOutput.vi"("error in (no error)"=w365, "Output"=1.0, "MotorControlDevRef"=w374) -> ("error out"=w403:errorcluster)  [unwired: 6 in, 2 out]
          n132 = call <vilib>:"WPI_MotorControlSetOutput.vi"("error in (no error)"=w403, "Output"=-1.0, "MotorControlDevRef"=w373) -> ("error out"=w402:errorcluster)  [unwired: 6 in, 2 out]
          n133 = call <vilib>:"WPI_RobotDriveDelayAndUpdateSafety.vi"("error in (no error)"=w402, "Delay (s)"=0.5, "RobotDriveDevRef"=w376) -> ()  [unwired: 7 in, 2 out]
        }
      }
    }
    frame "Alternative 1" {
      # "LEFT POSiTION"
      # "This sample code describes robot movements in an array. You can extend it to control other motors\non your robot. You can also use file I/O to move the data to a text file."
      n134 = case shown="\"L\"" w412 {
        tunnel: w411 -> [w416 w466]
        tunnel: w410 -> [w415 w465]
        tunnel: w409 -> [w414 w464]
        tunnel: w408 -> [w413 w467]
        tunnel: w407 -> [_ w444]
        tunnel: w406 -> [_ w434]
        frame "R", Default {
          n135 = call <vilib>:"WPI_RobotDriveTankDrive.vi"("error in (no error)"=w416, "Right axis value"=0.82 ("Y axis value"), "Left axis value"=0.8 ("X axis value"), "RobotDriveDevRef"=w413) -> ("error out"=w422:errorcluster, "RobotDriveDevRef"=w421:T3)  [unwired: 5 in, 1 out]
          n136 = call <vilib>:"WPI_RobotDriveDelayAndUpdateSafety.vi"("error in (no error)"=w422, "Delay (s)"=1.4, "RobotDriveDevRef"=w421) -> ("error out"=w430:errorcluster, "RobotDriveDevRef 2"=w429:T3)  [unwired: 7 in]
          n137 = call-poly <vilib>:"WPI_RobotDriveArcadeDrive.vi"("error in (no error)"=w430, "Y axis value"=0.0, "RobotDriveDevRef"=w429) -> ("error out"=w424:errorcluster, "RobotDriveDevRef"=w427:T3)  [unwired: 6 in, 1 out]
          n138 = call <vilib>:"WPI_MotorControlSetOutput.vi"("error in (no error)"=w424, "Output"=0.0, "MotorControlDevRef"=w415) -> ("error out"=w425:errorcluster)  [unwired: 6 in, 2 out]
          n139 = call <vilib>:"WPI_MotorControlSetOutput.vi"("error in (no error)"=w425, "Output"=0.0, "MotorControlDevRef"=w414) -> ("error out"=w423:errorcluster)  [unwired: 6 in, 2 out]
          n140 = call <vilib>:"WPI_RobotDriveDelayAndUpdateSafety.vi"("error in (no error)"=w423, "Delay (s)"=0.5, "RobotDriveDevRef"=w427) -> ()  [unwired: 7 in, 2 out]
        }
        frame "L" {
          n141 = call <vilib>:"WPI_RobotDriveTankDrive.vi"("error in (no error)"=w466, "Right axis value"=0.82 ("Y axis value"), "Left axis value"=0.8 ("X axis value"), "RobotDriveDevRef"=w467) -> ("error out"=w480:errorcluster, "RobotDriveDevRef"=w479:T3)  [unwired: 5 in, 1 out]
          n142 = call <vilib>:"WPI_RobotDriveDelayAndUpdateSafety.vi"("error in (no error)"=w480, "Delay (s)"=1.375, "RobotDriveDevRef"=w479) -> ("error out"=w468:errorcluster, "RobotDriveDevRef 2"=w469:T3)  [unwired: 7 in]
          n143 = call <vilib>:"WPI_RobotDriveTankDrive.vi"("error in (no error)"=w468, "Right axis value"=-0.85 ("Y axis value"), "Left axis value"=0.85 ("X axis value"), "RobotDriveDevRef"=w469) -> ("error out"=w473:errorcluster, "RobotDriveDevRef"=w472:T3)  [unwired: 5 in, 1 out]
          n144 = call <vilib>:"WPI_RobotDriveDelayAndUpdateSafety.vi"("error in (no error)"=w473, "Delay (s)"=0.35, "RobotDriveDevRef"=w472) -> ("error out"=w459:errorcluster, "RobotDriveDevRef 2"=w460:T3)  [unwired: 7 in]
          n145 = call-poly <vilib>:"WPI_RobotDriveArcadeDrive.vi"("error in (no error)"=w459, "Y axis value"=0.6, "RobotDriveDevRef"=w460) -> ("error out"=w456:errorcluster, "RobotDriveDevRef"=w457:T3)  [unwired: 6 in, 1 out]
          n146 = call <vilib>:"WPI_RobotDriveDelayAndUpdateSafety.vi"("error in (no error)"=w456, "Delay (s)"=0.8, "RobotDriveDevRef"=w457) -> ("error out"=w454:errorcluster, "RobotDriveDevRef 2"=w453:T3)  [unwired: 7 in]
          n147 = call-poly <vilib>:"WPI_RobotDriveArcadeDrive.vi"("error in (no error)"=w454, "Y axis value"=0.0, "X axis value"=0.0, "RobotDriveDevRef"=w453) -> ("error out"=w445:errorcluster, "RobotDriveDevRef"=w441:T3)  [unwired: 5 in, 1 out]
          n148 = call <vilib>:"WPI_MotorControlSetOutput.vi"("error in (no error)"=w445, "Output"=-1.0 ("Delay (s)"), "MotorControlDevRef"=w444) -> ("error out"=w440:errorcluster, "MotorControlDevRef"=w443:T4)  [unwired: 6 in, 1 out]
          n149 = call <vilib>:"WPI_RobotDriveDelayAndUpdateSafety.vi"("error in (no error)"=w440, "Delay (s)"=0.5, "RobotDriveDevRef"=w441) -> ("error out"=w437:errorcluster, "RobotDriveDevRef 2"=w438:T3)  [unwired: 7 in]
          n150 = call <vilib>:"WPI_MotorControlSetOutput.vi"("error in (no error)"=w437, "Output"=0.3 ("Delay (s)"), "MotorControlDevRef"=w434) -> ("error out"=w436:errorcluster)  [unwired: 6 in, 2 out]
          n151 = call <vilib>:"WPI_RobotDriveDelayAndUpdateSafety.vi"("error in (no error)"=w436, "Delay (s)"=0.05, "RobotDriveDevRef"=w438) -> ("error out"=w433:errorcluster, "RobotDriveDevRef 2"=w452:T3)  [unwired: 7 in]
          n152 = call-poly <vilib>:"WPI_RobotDriveArcadeDrive.vi"("error in (no error)"=w433, "Y axis value"=0.5, "RobotDriveDevRef"=w452) -> ("error out"=w447:errorcluster, "RobotDriveDevRef"=w484:T3)  [unwired: 6 in, 1 out]
          n153 = call <vilib>:"WPI_MotorControlSetOutput.vi"("error in (no error)"=w447, "Output"=0.0, "MotorControlDevRef"=w443) -> ("error out"=w446:errorcluster)  [unwired: 6 in, 2 out]
          n154 = call <vilib>:"WPI_MotorControlSetOutput.vi"("error in (no error)"=w446, "Output"=1.0, "MotorControlDevRef"=w465) -> ("error out"=w482:errorcluster)  [unwired: 6 in, 2 out]
          n155 = call <vilib>:"WPI_MotorControlSetOutput.vi"("error in (no error)"=w482, "Output"=-1.0, "MotorControlDevRef"=w464) -> ("error out"=w481:errorcluster)  [unwired: 6 in, 2 out]
          n156 = call <vilib>:"WPI_RobotDriveDelayAndUpdateSafety.vi"("error in (no error)"=w481, "Delay (s)"=0.5, "RobotDriveDevRef"=w484) -> ("error out"=w461:errorcluster, "RobotDriveDevRef 2"=w462:T3)  [unwired: 7 in]
          n157 = call-poly <vilib>:"WPI_RobotDriveArcadeDrive.vi"("error in (no error)"=w461, "Y axis value"=0.0, "RobotDriveDevRef"=w462) -> ()  [unwired: 6 in, 3 out]
        }
      }
    }
    frame "Alternative 2" {
      # "RIGHT POSiTION"
      # "This sample code describes robot movements in an array. You can extend it to control other motors\non your robot. You can also use file I/O to move the data to a text file."
      n158 = case shown="\"R\"" w492 {
        tunnel: w491 -> [w494 w527]
        tunnel: w490 -> [w495 w526]
        tunnel: w489 -> [w496 w525]
        tunnel: w488 -> [w493 w528]
        tunnel: w487 -> [_ w523]
        tunnel: w486 -> [_ w512]
        frame "L", Default {
          n159 = call <vilib>:"WPI_RobotDriveTankDrive.vi"("error in (no error)"=w494, "Right axis value"=0.82 ("Y axis value"), "Left axis value"=0.8 ("X axis value"), "RobotDriveDevRef"=w493) -> ("error out"=w502:errorcluster, "RobotDriveDevRef"=w501:T3)  [unwired: 5 in, 1 out]
          n160 = call <vilib>:"WPI_RobotDriveDelayAndUpdateSafety.vi"("error in (no error)"=w502, "Delay (s)"=1.4, "RobotDriveDevRef"=w501) -> ("error out"=w510:errorcluster, "RobotDriveDevRef 2"=w509:T3)  [unwired: 7 in]
          n161 = call-poly <vilib>:"WPI_RobotDriveArcadeDrive.vi"("error in (no error)"=w510, "Y axis value"=0.0, "RobotDriveDevRef"=w509) -> ("error out"=w504:errorcluster, "RobotDriveDevRef"=w507:T3)  [unwired: 6 in, 1 out]
          n162 = call <vilib>:"WPI_MotorControlSetOutput.vi"("error in (no error)"=w504, "Output"=0.0, "MotorControlDevRef"=w495) -> ("error out"=w505:errorcluster)  [unwired: 6 in, 2 out]
          n163 = call <vilib>:"WPI_MotorControlSetOutput.vi"("error in (no error)"=w505, "Output"=0.0, "MotorControlDevRef"=w496) -> ("error out"=w503:errorcluster)  [unwired: 6 in, 2 out]
          n164 = call <vilib>:"WPI_RobotDriveDelayAndUpdateSafety.vi"("error in (no error)"=w503, "Delay (s)"=0.5, "RobotDriveDevRef"=w507) -> ()  [unwired: 7 in, 2 out]
        }
        frame "R" {
          n165 = call <vilib>:"WPI_RobotDriveTankDrive.vi"("error in (no error)"=w527, "Right axis value"=0.82 ("Y axis value"), "Left axis value"=0.8 ("X axis value"), "RobotDriveDevRef"=w528) -> ("error out"=w559:errorcluster, "RobotDriveDevRef"=w558:T3)  [unwired: 5 in, 1 out]
          n166 = call <vilib>:"WPI_RobotDriveDelayAndUpdateSafety.vi"("error in (no error)"=w559, "Delay (s)"=1.375, "RobotDriveDevRef"=w558) -> ("error out"=w547:errorcluster, "RobotDriveDevRef 2"=w548:T3)  [unwired: 7 in]
          n167 = call <vilib>:"WPI_RobotDriveTankDrive.vi"("error in (no error)"=w547, "Right axis value"=0.85 ("Y axis value"), "Left axis value"=-0.85 ("X axis value"), "RobotDriveDevRef"=w548) -> ("error out"=w552:errorcluster, "RobotDriveDevRef"=w551:T3)  [unwired: 5 in, 1 out]
          n168 = call <vilib>:"WPI_RobotDriveDelayAndUpdateSafety.vi"("error in (no error)"=w552, "Delay (s)"=0.35, "RobotDriveDevRef"=w551) -> ("error out"=w542:errorcluster, "RobotDriveDevRef 2"=w543:T3)  [unwired: 7 in]
          n169 = call-poly <vilib>:"WPI_RobotDriveArcadeDrive.vi"("error in (no error)"=w542, "Y axis value"=0.6, "RobotDriveDevRef"=w543) -> ("error out"=w539:errorcluster, "RobotDriveDevRef"=w540:T3)  [unwired: 6 in, 1 out]
          n170 = call <vilib>:"WPI_RobotDriveDelayAndUpdateSafety.vi"("error in (no error)"=w539, "Delay (s)"=0.8, "RobotDriveDevRef"=w540) -> ("error out"=w537:errorcluster, "RobotDriveDevRef 2"=w536:T3)  [unwired: 7 in]
          n171 = call-poly <vilib>:"WPI_RobotDriveArcadeDrive.vi"("error in (no error)"=w537, "Y axis value"=0.0, "X axis value"=0.0, "RobotDriveDevRef"=w536) -> ("error out"=w524:errorcluster, "RobotDriveDevRef"=w518:T3)  [unwired: 5 in, 1 out]
          n172 = call <vilib>:"WPI_MotorControlSetOutput.vi"("error in (no error)"=w524, "Output"=-1.0 ("Delay (s)"), "MotorControlDevRef"=w523) -> ("error out"=w521:errorcluster, "MotorControlDevRef"=w522:T4)  [unwired: 6 in, 1 out]
          n173 = call <vilib>:"WPI_RobotDriveDelayAndUpdateSafety.vi"("error in (no error)"=w521, "Delay (s)"=0.5, "RobotDriveDevRef"=w518) -> ("error out"=w520:errorcluster, "RobotDriveDevRef 2"=w517:T3)  [unwired: 7 in]
          n174 = call <vilib>:"WPI_MotorControlSetOutput.vi"("error in (no error)"=w520, "Output"=0.3 ("Delay (s)"), "MotorControlDevRef"=w512) -> ("error out"=w519:errorcluster)  [unwired: 6 in, 2 out]
          n175 = call <vilib>:"WPI_RobotDriveDelayAndUpdateSafety.vi"("error in (no error)"=w519, "Delay (s)"=0.05, "RobotDriveDevRef"=w517) -> ("error out"=w513:errorcluster, "RobotDriveDevRef 2"=w535:T3)  [unwired: 7 in]
          n176 = call-poly <vilib>:"WPI_RobotDriveArcadeDrive.vi"("error in (no error)"=w513, "Y axis value"=0.5, "RobotDriveDevRef"=w535) -> ("error out"=w530:errorcluster, "RobotDriveDevRef"=w563:T3)  [unwired: 6 in, 1 out]
          n177 = call <vilib>:"WPI_MotorControlSetOutput.vi"("error in (no error)"=w530, "Output"=0.0, "MotorControlDevRef"=w522) -> ("error out"=w529:errorcluster)  [unwired: 6 in, 2 out]
          n178 = call <vilib>:"WPI_MotorControlSetOutput.vi"("error in (no error)"=w529, "Output"=1.0, "MotorControlDevRef"=w526) -> ("error out"=w561:errorcluster)  [unwired: 6 in, 2 out]
          n179 = call <vilib>:"WPI_MotorControlSetOutput.vi"("error in (no error)"=w561, "Output"=-1.0, "MotorControlDevRef"=w525) -> ("error out"=w560:errorcluster)  [unwired: 6 in, 2 out]
          n180 = call <vilib>:"WPI_RobotDriveDelayAndUpdateSafety.vi"("error in (no error)"=w560, "Delay (s)"=0.5, "RobotDriveDevRef"=w563) -> ("error out"=w544:errorcluster, "RobotDriveDevRef 2"=w545:T3)  [unwired: 7 in]
          n181 = call-poly <vilib>:"WPI_RobotDriveArcadeDrive.vi"("error in (no error)"=w544, "Y axis value"=0.0, "RobotDriveDevRef"=w545) -> ()  [unwired: 6 in, 3 out]
        }
      }
    }
    frame "null" {
      n182 = call <vilib>:"WPI_RobotDriveTankDrive.vi"("error in (no error)"=w575, "Right axis value"=0.82, "Left axis value"=0.8 ("Output"), "RobotDriveDevRef"=w576) -> ("error out"=w578:errorcluster, "RobotDriveDevRef"=w577:T3)  [unwired: 5 in, 1 out]
      n183 = call <vilib>:"WPI_RobotDriveDelayAndUpdateSafety.vi"("error in (no error)"=w578, "Delay (s)"=3.0 ("Output"), "RobotDriveDevRef"=w577) -> ("error out"=w574:errorcluster, "RobotDriveDevRef 2"=w573:T3)  [unwired: 7 in]
      n184 = call <vilib>:"WPI_RobotDriveTankDrive.vi"("error in (no error)"=w574, "Left axis value"=0.0 ("Output"), "RobotDriveDevRef"=w573) -> ("error out"=w572:errorcluster, "RobotDriveDevRef"=w571:T3)  [unwired: 6 in, 1 out]
      n185 = call <vilib>:"WPI_RobotDriveDelayAndUpdateSafety.vi"("error in (no error)"=w572, "Delay (s)"=0.1 ("Output"), "RobotDriveDevRef"=w571) -> ()  [unwired: 7 in, 2 out]
    }
    frame "scaleR" {
      n186 = case shown="\"LR\", \"RR\", Default" w587 {
        tunnel: w586 -> [w657 w671]
        tunnel: w585 -> [w637 w669]
        tunnel: w584 -> [w638 w670]
        tunnel: w583 -> [w634 _]
        tunnel: w582 -> [w633 _]
        tunnel: w581 -> [w632 _]
        tunnel: w580 -> [_ w672]
        tunnel: w579 -> [w601 _]
        frame "LR", "RR", Default {
          # "300in to scale"
          n187 = call <vilib>:"WPI_SwitchGetLimitValue.vi"("error in (no error)"=w634, "SwitchDevRef"=w633) -> ("Switch Pressed"=w635:bool)  [unwired: 7 in, 2 out]
          n188 = call <vilib>:"WPI_RobotDriveTankDrive.vi"("Right axis value"=0.82 ("Y axis value"), "Left axis value"=0.8 ("X axis value"), "RobotDriveDevRef"=w657) -> ("error out"=w663:errorcluster, "RobotDriveDevRef"=w662:T3)  [unwired: 6 in, 1 out]
          n189 = case shown="False" w635 {
            tunnel: [-0.65 ("Output") 0.0 ("Output")] -> w636
            frame False {
            }
            frame True {
            }
          }
          n190 = call <vilib>:"WPI_RobotDriveDelayAndUpdateSafety.vi"("error in (no error)"=w663, "Delay (s)"=3.5, "RobotDriveDevRef"=w662) -> ("error out"=w655:errorcluster, "RobotDriveDevRef 2"=w656:T3)  [unwired: 7 in]
          n191 = call <vilib>:"WPI_RobotDriveTankDrive.vi"("error in (no error)"=w655, "Right axis value"=0.0, "Left axis value"=0.0, "RobotDriveDevRef"=w656) -> ("error out"=w652:errorcluster, "RobotDriveDevRef"=w650:T3)  [unwired: 5 in, 1 out]
          n192 = call <vilib>:"WPI_MotorControlSetOutput.vi"("error in (no error)"=w652, "Output"=w636, "MotorControlDevRef"=w632) -> ("error out"=w649:errorcluster, "MotorControlDevRef"=w631:T4)  [unwired: 6 in, 1 out]
          n193 = call <vilib>:"WPI_RobotDriveDelayAndUpdateSafety.vi"("error in (no error)"=w649, "Delay (s)"=2.0, "RobotDriveDevRef"=w650) -> ("error out"=w643:errorcluster, "RobotDriveDevRef 2"=w644:T3)  [unwired: 7 in]
          n194 = call <vilib>:"WPI_RobotDriveTankDrive.vi"("error in (no error)"=w643, "Right axis value"=0.6, "Left axis value"=0.0, "RobotDriveDevRef"=w644) -> ("error out"=w630:errorcluster, "RobotDriveDevRef"=w645:T3)  [unwired: 5 in, 1 out]
          n195 = call <vilib>:"WPI_MotorControlSetOutput.vi"("error in (no error)"=w630, "Output"=0.0, "MotorControlDevRef"=w631) -> ("error out"=w604:errorcluster)  [unwired: 6 in, 2 out]
          n196 = call <vilib>:"WPI_RobotDriveDelayAndUpdateSafety.vi"("error in (no error)"=w604, "Delay (s)"=1.2, "RobotDriveDevRef"=w645) -> ("error out"=w639:errorcluster, "RobotDriveDevRef 2"=w640:T3)  [unwired: 7 in]
          n197 = call <vilib>:"WPI_RobotDriveTankDrive.vi"("error in (no error)"=w639, "Right axis value"=0.0, "Left axis value"=0.0, "RobotDriveDevRef"=w640) -> ("error out"=w603:errorcluster, "RobotDriveDevRef"=w615:T3)  [unwired: 5 in, 1 out]
          n198 = call <vilib>:"WPI_MotorControlSetOutput.vi"("error in (no error)"=w603, "Output"=0.1, "MotorControlDevRef"=w601) -> ("error out"=w602:errorcluster, "MotorControlDevRef"=w593:T4)  [unwired: 6 in, 1 out]
          n199 = call <vilib>:"WPI_RobotDriveDelayAndUpdateSafety.vi"("error in (no error)"=w602, "Delay (s)"=0.025, "RobotDriveDevRef"=w615) -> ("error out"=w594:errorcluster, "RobotDriveDevRef 2"=w595:T3)  [unwired: 7 in]
          n200 = call <vilib>:"WPI_RobotDriveTankDrive.vi"("error in (no error)"=w594, "Right axis value"=0.0, "Left axis value"=0.0, "RobotDriveDevRef"=w595) -> ("error out"=w591:errorcluster, "RobotDriveDevRef"=w598:T3)  [unwired: 5 in, 1 out]
          n201 = call <vilib>:"WPI_MotorControlSetOutput.vi"("error in (no error)"=w591, "Output"=0.0, "MotorControlDevRef"=w593) -> ("error out"=w590:errorcluster)  [unwired: 6 in, 2 out]
          n202 = call <vilib>:"WPI_RobotDriveDelayAndUpdateSafety.vi"("error in (no error)"=w590, "Delay (s)"=0.1, "RobotDriveDevRef"=w598) -> ("error out"=w588:errorcluster, "RobotDriveDevRef 2"=w589:T3)  [unwired: 7 in]
          n203 = call <vilib>:"WPI_RobotDriveTankDrive.vi"("error in (no error)"=w588, "Right axis value"=0.0, "Left axis value"=0.0, "RobotDriveDevRef"=w589) -> ("error out"=w614:errorcluster, "RobotDriveDevRef"=w613:T3)  [unwired: 5 in, 1 out]
          n204 = call <vilib>:"WPI_MotorControlSetOutput.vi"("error in (no error)"=w614, "Output"=1.0, "MotorControlDevRef"=w638) -> ("error out"=w665:errorcluster, "MotorControlDevRef"=w622:T4)  [unwired: 6 in, 1 out]
          n205 = call <vilib>:"WPI_MotorControlSetOutput.vi"("error in (no error)"=w665, "Output"=-1.0, "MotorControlDevRef"=w637) -> ("error out"=w664:errorcluster, "MotorControlDevRef"=w621:T4)  [unwired: 6 in, 1 out]
          n206 = call <vilib>:"WPI_RobotDriveDelayAndUpdateSafety.vi"("error in (no error)"=w664, "Delay (s)"=0.5, "RobotDriveDevRef"=w613) -> ("error out"=w625:errorcluster, "RobotDriveDevRef 2"=w626:T3)  [unwired: 7 in]
          n207 = call <vilib>:"WPI_RobotDriveTankDrive.vi"("error in (no error)"=w625, "Right axis value"=-0.5, "Left axis value"=-0.5, "RobotDriveDevRef"=w626) -> ("error out"=w623:errorcluster, "RobotDriveDevRef"=w610:T3)  [unwired: 5 in, 1 out]
          n208 = call <vilib>:"WPI_MotorControlSetOutput.vi"("error in (no error)"=w623, "Output"=0.0, "MotorControlDevRef"=w622) -> ("error out"=w624:errorcluster)  [unwired: 6 in, 2 out]
          n209 = call <vilib>:"WPI_MotorControlSetOutput.vi"("error in (no error)"=w624, "Output"=0.0, "MotorControlDevRef"=w621) -> ("error out"=w609:errorcluster)  [unwired: 6 in, 2 out]
          n210 = call <vilib>:"WPI_RobotDriveDelayAndUpdateSafety.vi"("error in (no error)"=w609, "Delay (s)"=1.5, "RobotDriveDevRef"=w610) -> ("error out"=w605:errorcluster, "RobotDriveDevRef 2"=w606:T3)  [unwired: 7 in]
          n211 = call <vilib>:"WPI_RobotDriveTankDrive.vi"("error in (no error)"=w605, "Right axis value"=0.0, "Left axis value"=0.0, "RobotDriveDevRef"=w606) -> ()  [unwired: 5 in, 3 out]
        }
        frame "LL", "RL" {
          n212 = call <vilib>:"WPI_RobotDriveTankDrive.vi"("error in (no error)"=w672, "Right axis value"=0.82 ("Y axis value"), "Left axis value"=0.8 ("X axis value"), "RobotDriveDevRef"=w671) -> ("error out"=w678:errorcluster, "RobotDriveDevRef"=w677:T3)  [unwired: 5 in, 1 out]
          n213 = call <vilib>:"WPI_RobotDriveDelayAndUpdateSafety.vi"("error in (no error)"=w678, "Delay (s)"=1.4, "RobotDriveDevRef"=w677) -> ("error out"=w686:errorcluster, "RobotDriveDevRef 2"=w685:T3)  [unwired: 7 in]
          n214 = call-poly <vilib>:"WPI_RobotDriveArcadeDrive.vi"("error in (no error)"=w686, "Y axis value"=0.0, "RobotDriveDevRef"=w685) -> ("error out"=w680:errorcluster, "RobotDriveDevRef"=w683:T3)  [unwired: 6 in, 1 out]
          n215 = call <vilib>:"WPI_MotorControlSetOutput.vi"("error in (no error)"=w680, "Output"=0.0, "MotorControlDevRef"=w670) -> ("error out"=w681:errorcluster)  [unwired: 6 in, 2 out]
          n216 = call <vilib>:"WPI_MotorControlSetOutput.vi"("error in (no error)"=w681, "Output"=0.0, "MotorControlDevRef"=w669) -> ("error out"=w679:errorcluster)  [unwired: 6 in, 2 out]
          n217 = call <vilib>:"WPI_RobotDriveDelayAndUpdateSafety.vi"("error in (no error)"=w679, "Delay (s)"=0.5, "RobotDriveDevRef"=w683) -> ()  [unwired: 7 in, 2 out]
        }
      }
    }
    frame "SF" {
    }
    frame "scale L" {
      n218 = case shown="\"LL\", \"RL\", Default" w696 {
        tunnel: w695 -> [w766 w780]
        tunnel: w694 -> [w746 w778]
        tunnel: w693 -> [w747 w779]
        tunnel: w692 -> [w743 _]
        tunnel: w691 -> [w742 _]
        tunnel: w690 -> [w741 _]
        tunnel: w689 -> [_ w781]
        tunnel: w688 -> [w710 _]
        frame "LL", "RL", Default {
          # "300in to scale"
          n219 = call <vilib>:"WPI_SwitchGetLimitValue.vi"("error in (no error)"=w743, "SwitchDevRef"=w742) -> ("Switch Pressed"=w744:bool)  [unwired: 7 in, 2 out]
          n220 = call <vilib>:"WPI_RobotDriveTankDrive.vi"("Right axis value"=0.82 ("Y axis value"), "Left axis value"=0.8 ("X axis value"), "RobotDriveDevRef"=w766) -> ("error out"=w772:errorcluster, "RobotDriveDevRef"=w771:T3)  [unwired: 6 in, 1 out]
          n221 = case shown="False" w744 {
            tunnel: [-0.65 ("Output") 0.0 ("Output")] -> w745
            frame False {
            }
            frame True {
            }
          }
          n222 = call <vilib>:"WPI_RobotDriveDelayAndUpdateSafety.vi"("error in (no error)"=w772, "Delay (s)"=3.5, "RobotDriveDevRef"=w771) -> ("error out"=w764:errorcluster, "RobotDriveDevRef 2"=w765:T3)  [unwired: 7 in]
          n223 = call <vilib>:"WPI_RobotDriveTankDrive.vi"("error in (no error)"=w764, "Right axis value"=0.0, "Left axis value"=0.0, "RobotDriveDevRef"=w765) -> ("error out"=w761:errorcluster, "RobotDriveDevRef"=w759:T3)  [unwired: 5 in, 1 out]
          n224 = call <vilib>:"WPI_MotorControlSetOutput.vi"("error in (no error)"=w761, "Output"=w745, "MotorControlDevRef"=w741) -> ("error out"=w758:errorcluster, "MotorControlDevRef"=w740:T4)  [unwired: 6 in, 1 out]
          n225 = call <vilib>:"WPI_RobotDriveDelayAndUpdateSafety.vi"("error in (no error)"=w758, "Delay (s)"=2.0, "RobotDriveDevRef"=w759) -> ("error out"=w752:errorcluster, "RobotDriveDevRef 2"=w753:T3)  [unwired: 7 in]
          n226 = call <vilib>:"WPI_RobotDriveTankDrive.vi"("error in (no error)"=w752, "Right axis value"=0.0, "Left axis value"=0.6, "RobotDriveDevRef"=w753) -> ("error out"=w739:errorcluster, "RobotDriveDevRef"=w754:T3)  [unwired: 5 in, 1 out]
          n227 = call <vilib>:"WPI_MotorControlSetOutput.vi"("error in (no error)"=w739, "Output"=0.0, "MotorControlDevRef"=w740) -> ("error out"=w713:errorcluster)  [unwired: 6 in, 2 out]
          n228 = call <vilib>:"WPI_RobotDriveDelayAndUpdateSafety.vi"("error in (no error)"=w713, "Delay (s)"=1.2, "RobotDriveDevRef"=w754) -> ("error out"=w748:errorcluster, "RobotDriveDevRef 2"=w749:T3)  [unwired: 7 in]
          n229 = call <vilib>:"WPI_RobotDriveTankDrive.vi"("error in (no error)"=w748, "Right axis value"=0.0, "Left axis value"=0.0, "RobotDriveDevRef"=w749) -> ("error out"=w712:errorcluster, "RobotDriveDevRef"=w724:T3)  [unwired: 5 in, 1 out]
          n230 = call <vilib>:"WPI_MotorControlSetOutput.vi"("error in (no error)"=w712, "Output"=0.1, "MotorControlDevRef"=w710) -> ("error out"=w711:errorcluster, "MotorControlDevRef"=w702:T4)  [unwired: 6 in, 1 out]
          n231 = call <vilib>:"WPI_RobotDriveDelayAndUpdateSafety.vi"("error in (no error)"=w711, "Delay (s)"=0.025, "RobotDriveDevRef"=w724) -> ("error out"=w703:errorcluster, "RobotDriveDevRef 2"=w704:T3)  [unwired: 7 in]
          n232 = call <vilib>:"WPI_RobotDriveTankDrive.vi"("error in (no error)"=w703, "Right axis value"=0.0, "Left axis value"=0.0, "RobotDriveDevRef"=w704) -> ("error out"=w700:errorcluster, "RobotDriveDevRef"=w707:T3)  [unwired: 5 in, 1 out]
          n233 = call <vilib>:"WPI_MotorControlSetOutput.vi"("error in (no error)"=w700, "Output"=0.0, "MotorControlDevRef"=w702) -> ("error out"=w699:errorcluster)  [unwired: 6 in, 2 out]
          n234 = call <vilib>:"WPI_RobotDriveDelayAndUpdateSafety.vi"("error in (no error)"=w699, "Delay (s)"=0.1, "RobotDriveDevRef"=w707) -> ("error out"=w697:errorcluster, "RobotDriveDevRef 2"=w698:T3)  [unwired: 7 in]
          n235 = call <vilib>:"WPI_RobotDriveTankDrive.vi"("error in (no error)"=w697, "Right axis value"=0.0, "Left axis value"=0.0, "RobotDriveDevRef"=w698) -> ("error out"=w723:errorcluster, "RobotDriveDevRef"=w722:T3)  [unwired: 5 in, 1 out]
          n236 = call <vilib>:"WPI_MotorControlSetOutput.vi"("error in (no error)"=w723, "Output"=1.0, "MotorControlDevRef"=w747) -> ("error out"=w774:errorcluster, "MotorControlDevRef"=w731:T4)  [unwired: 6 in, 1 out]
          n237 = call <vilib>:"WPI_MotorControlSetOutput.vi"("error in (no error)"=w774, "Output"=-1.0, "MotorControlDevRef"=w746) -> ("error out"=w773:errorcluster, "MotorControlDevRef"=w730:T4)  [unwired: 6 in, 1 out]
          n238 = call <vilib>:"WPI_RobotDriveDelayAndUpdateSafety.vi"("error in (no error)"=w773, "Delay (s)"=0.5, "RobotDriveDevRef"=w722) -> ("error out"=w734:errorcluster, "RobotDriveDevRef 2"=w735:T3)  [unwired: 7 in]
          n239 = call <vilib>:"WPI_RobotDriveTankDrive.vi"("error in (no error)"=w734, "Right axis value"=-0.5, "Left axis value"=-0.5, "RobotDriveDevRef"=w735) -> ("error out"=w732:errorcluster, "RobotDriveDevRef"=w719:T3)  [unwired: 5 in, 1 out]
          n240 = call <vilib>:"WPI_MotorControlSetOutput.vi"("error in (no error)"=w732, "Output"=0.0, "MotorControlDevRef"=w731) -> ("error out"=w733:errorcluster)  [unwired: 6 in, 2 out]
          n241 = call <vilib>:"WPI_MotorControlSetOutput.vi"("error in (no error)"=w733, "Output"=0.0, "MotorControlDevRef"=w730) -> ("error out"=w718:errorcluster)  [unwired: 6 in, 2 out]
          n242 = call <vilib>:"WPI_RobotDriveDelayAndUpdateSafety.vi"("error in (no error)"=w718, "Delay (s)"=1.5, "RobotDriveDevRef"=w719) -> ("error out"=w714:errorcluster, "RobotDriveDevRef 2"=w715:T3)  [unwired: 7 in]
          n243 = call <vilib>:"WPI_RobotDriveTankDrive.vi"("error in (no error)"=w714, "Right axis value"=0.0, "Left axis value"=0.0, "RobotDriveDevRef"=w715) -> ()  [unwired: 5 in, 3 out]
        }
        frame "LRL", "RRR" {
          n244 = call <vilib>:"WPI_RobotDriveTankDrive.vi"("error in (no error)"=w781, "Right axis value"=0.82 ("Y axis value"), "Left axis value"=0.8 ("X axis value"), "RobotDriveDevRef"=w780) -> ("error out"=w787:errorcluster, "RobotDriveDevRef"=w786:T3)  [unwired: 5 in, 1 out]
          n245 = call <vilib>:"WPI_RobotDriveDelayAndUpdateSafety.vi"("error in (no error)"=w787, "Delay (s)"=1.4, "RobotDriveDevRef"=w786) -> ("error out"=w795:errorcluster, "RobotDriveDevRef 2"=w794:T3)  [unwired: 7 in]
          n246 = call-poly <vilib>:"WPI_RobotDriveArcadeDrive.vi"("error in (no error)"=w795, "Y axis value"=0.0, "RobotDriveDevRef"=w794) -> ("error out"=w789:errorcluster, "RobotDriveDevRef"=w792:T3)  [unwired: 6 in, 1 out]
          n247 = call <vilib>:"WPI_MotorControlSetOutput.vi"("error in (no error)"=w789, "Output"=0.0, "MotorControlDevRef"=w779) -> ("error out"=w790:errorcluster)  [unwired: 6 in, 2 out]
          n248 = call <vilib>:"WPI_MotorControlSetOutput.vi"("error in (no error)"=w790, "Output"=0.0, "MotorControlDevRef"=w778) -> ("error out"=w788:errorcluster)  [unwired: 6 in, 2 out]
          n249 = call <vilib>:"WPI_RobotDriveDelayAndUpdateSafety.vi"("error in (no error)"=w788, "Delay (s)"=0.5, "RobotDriveDevRef"=w792) -> ()  [unwired: 7 in, 2 out]
        }
      }
    }
  }
